vi "01 Maintenance.vi"() -> ()   [LabVIEW 2025]
doc: "This vi provides template for the front panel size fixing for GUI developement."
uses:
  Controls/Maintenance AO Cluster.ctl
  Host Globals/Global 1.vi
  <vilib>/FPGAPlugInAG/Dynamic/niLvFpga_Abort_Dynamic.vi
  <vilib>/FPGAPlugInAG/Dynamic/niLvFpga_Close_Dynamic.vi
  <vilib>/Utility/xml.llb/Read From XML File(string).vi
  <vilib>/rvi/interface/nirviMethod/nirviMethod.xnode
  <vilib>/rvi/interface/nirviCloseFPGA/nirviCloseFPGA.xnode
  <vilib>/rvi/interface/nirviOpenFPGA/nirviOpenFPGA.xnode
  <vilib>/FPGAPlugInAG/Dynamic/niLvFpga_Reset_Dynamic.vi
  <vilib>/FPGAPlugInAG/Dynamic/niLvFpga_Run_Dynamic.vi
  <vilib>/rvi/interface/nirviReadWriteControl/nirviReadWriteControl.xnode
  <vilib>/rvi/interface/Simulation/niFpgaSimulationCallBeginRW.vi
  <vilib>/rvi/errors/niLvFpgaAdjustHostInterfaceError.vi
  FPGA Bitfiles/old.lvbitx
  FPGA Bitfiles/oldMAINFPGANI9148_MKQg3WTXJXE.lvbitx
  NiFpgaLv.dll
panel:
  in  "Misc_P 2":T1={"Gain"=1.0, "offset"=0.0}
  in  "Intercooler_Out_P 2":T1={"Gain"=1.0, "offset"=0.0}
  in  "Intercooler_In_P 2":T1={"Gain"=1.0, "offset"=0.0}
  in  "Oil_P 2":T1={"Gain"=1.0, "offset"=0.0}
  in  "Exhaust_P 2":T1={"Gain"=1.0, "offset"=0.0}
  in  "Coolant_Out_P 2":T1={"Gain"=1.0, "offset"=0.0}
  in  "Coolant_In_P 2":T1={"Gain"=1.0, "offset"=0.0}
  out "Time":string
  out "User":string
  in  "Home Button":bool
  in  "Home":bool caption="Back"
  in  "Tab Control":T2(tab)
  in  "AO Cluster":T3
  in  "4":cluster{"Offset":dbl, "Gain":dbl}
  in  "6":cluster{"Offset":dbl, "Gain":dbl}
  in  "5":cluster{"Offset":dbl, "Gain":dbl}
  in  "2":cluster{"Offset":dbl, "Gain":dbl}
  in  "3":cluster{"Offset":dbl, "Gain":dbl}
  out "ANALOG INPUT":string[][](table)=[["5"], ["1"], ["2.5"], ["5"], ["85"], ["55"], ["7"], ["2"], ["4"], ["2"], ["4"], ["2"], ["5"], ["12.5"], ["22.5"], ["5.02"], ["22.8"], ["7"], ["5"], ["0"], ["0"], ["0.00"], ["0.2"], ["0.1"], ["0.2"]]
  in  "1":cluster{"Offset":dbl, "Gain":dbl}
  in  "DO Cluster":T4
  out "DI Cluster":T5
  # "MAINTENANCE"
  # "Parameters Name"
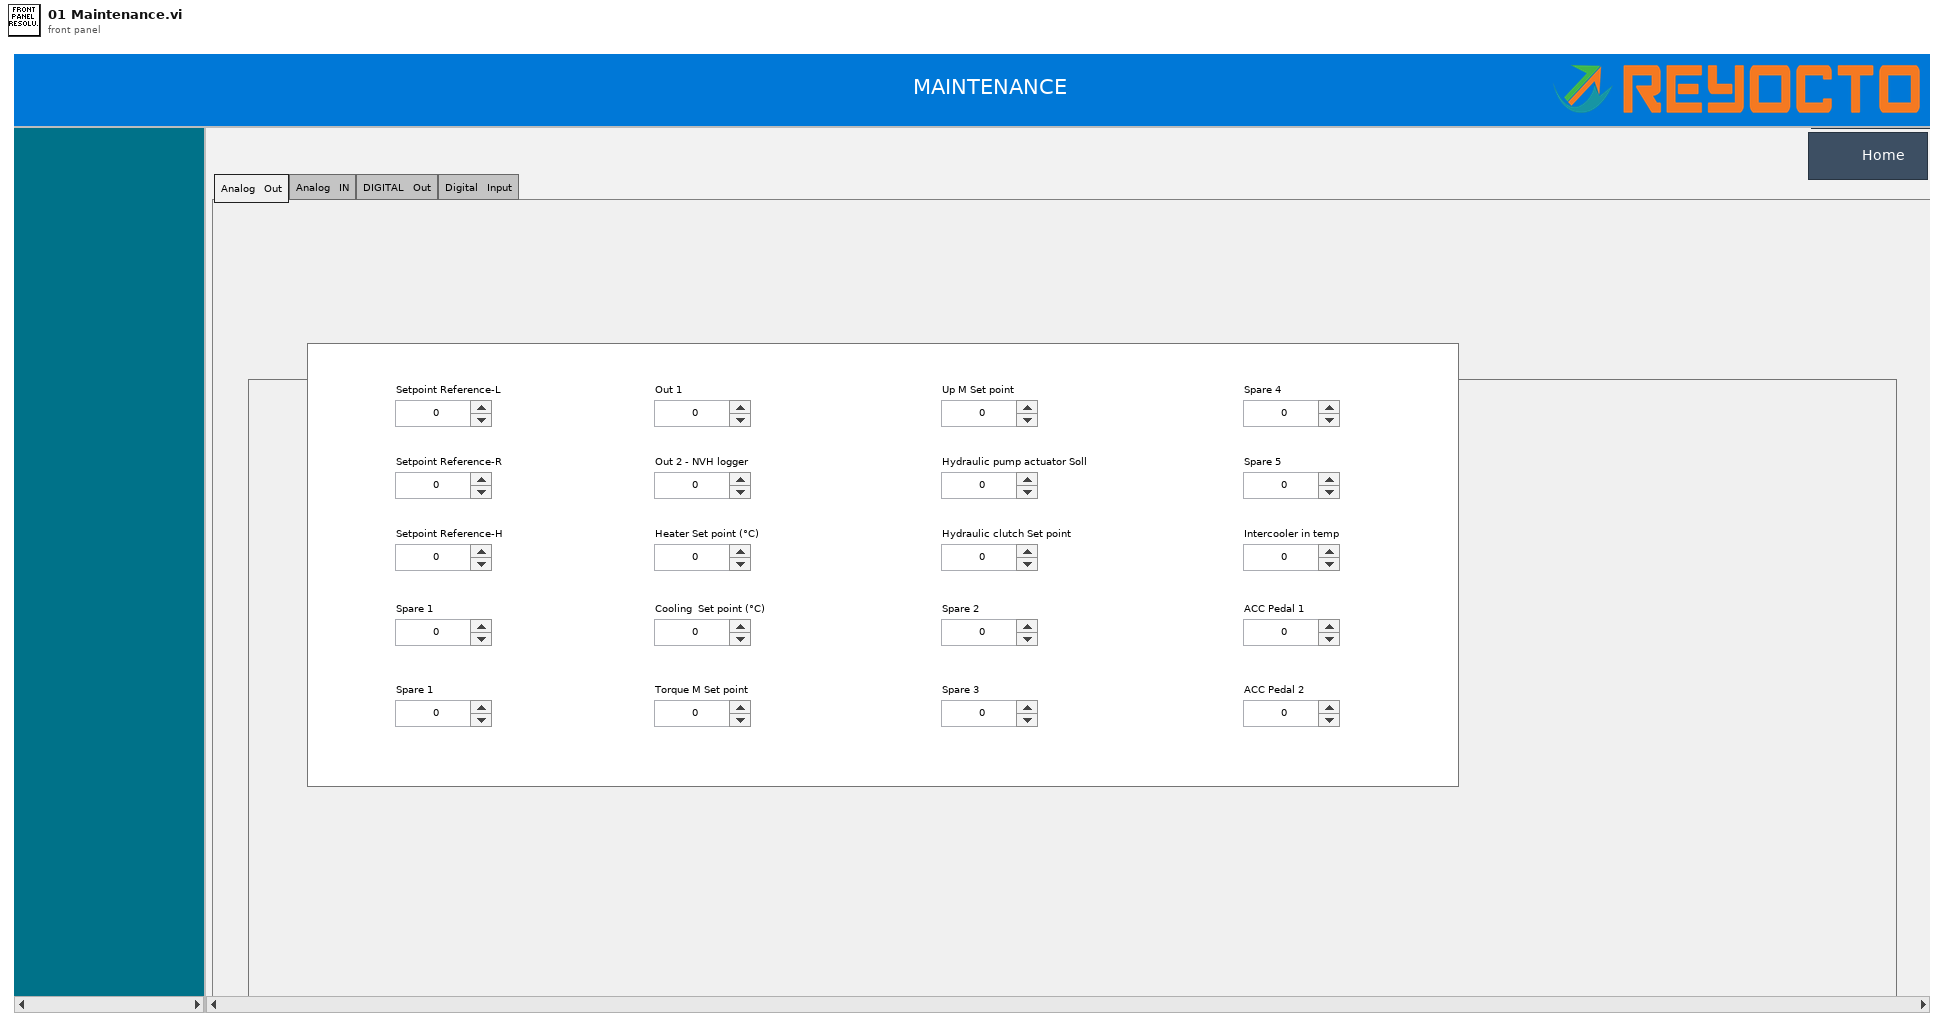
[diagram p1: front panel]
types:
  T1 = cluster{"Gain":fxp<+/-,24,5>, "offset":fxp<+/-,24,5>}
  T2 = enum32{"Analog   Out", "Analog   IN", "DIGITAL   Out", "Digital   Input"}
  T3 = typedef "Maintenance AO Cluster.ctl" = cluster{"AO 1":dbl, "AO 2":dbl, "AO 3":dbl, "AO 4":dbl, "AO 5":dbl, "AO 6":dbl, "AO 7":dbl, "AO 8":dbl, "AO 9":dbl, "AO 10":dbl, "AO 11":dbl, "AO 12":dbl, "AO 13":dbl, "AO 14":dbl, "AO 15":dbl, "AO 16":dbl, "AO 17":dbl, "AO 18":dbl, "AO 19":dbl, "AO 20":dbl}
  T4 = cluster{"0":bool, "1":bool, "2":bool, "3":bool, "4":bool, "5":bool, "6":bool, "7":bool, "8":bool, "9":bool, "10":bool, "11":bool, "12":bool, "13":bool, "14":bool, "15":bool, "16":bool, "17":bool, "18":bool, "19":bool, "20":bool, "21":bool, "22":bool, "23":bool, "24":bool, "25":bool, "26":bool, "27":bool, "28":bool, "29":bool, "30":bool, "31":bool, "32":bool, "33":bool, "34":bool, "35":bool, "36":bool, "37":bool, "38":bool, "39":bool, "40":bool, "41":bool, "42":bool, "43":bool, "44":bool, "45":bool, "46":bool, "47":bool, "48":bool, "49":bool, "50":bool, "51":bool, "52":bool, "53":bool, "54":bool, "55":bool, "56":bool, "57":bool, "58":bool, "59":bool, "60":bool, "61":bool, "62":bool, "63":bool}
  T5 = cluster{"1":bool, "2":bool, "3":bool, "4":bool, "5":bool, "6":bool, "7":bool, "8":bool, "9":bool, "10":bool, "11":bool, "12":bool, "13":bool, "14":bool, "15":bool, "16":bool, "17":bool, "18":bool, "19":bool, "20":bool, "21":bool, "22":bool, "23":bool, "24":bool, "25":bool, "26":bool, "27":bool, "28":bool, "29":bool, "30":bool, "31":bool, "32":bool, "33":bool, "34":bool, "35":bool, "36":bool, "37":bool, "38":bool, "39":bool, "40":bool, "41":bool, "42":bool, "43":bool, "44":bool, "45":bool, "46":bool, "47":bool, "48":bool, "49":bool, "50":bool, "51":bool, "52":bool, "53":bool, "54":bool, "55":bool, "56":bool, "57":bool, "58":bool, "59":bool, "60":bool, "61":bool, "62":bool, "63":bool, "64":bool}
  T6 = enum32{"invalid app kind", "Development System", "Run Time System", "Student Edition", "Embedded LabVIEW", "Evaluation", "Custom"}
  T7 = enum32{"Invalid", "Standard", "Closed", "Hidden", "Minimized", "Maximized"}
  T8 = cluster{"Core":cluster{"Current VI Reference":refnum<vi>, "Close Panel on Exit?":bool}, "AI Config path":path, "AO Config path":path, "DI Config path":path, "DO COnfig path":path, "AO Cluster":refnum<vi>, "DO Cluster":refnum<vi>, "DI Cluster":refnum<vi>, "Data":cluster{"Digital Output":refnum<k21>, "Set 1 DO":u32, "Maintenance":refnum<k21>, "Digital Input":refnum<k21>}, "Analog Data":string[][], "FPGA VI Reference Out":refnum<k20>, "FPGA VI Reference Out":refnum<k20>}
  T9 = cluster{"Digital Output":refnum<k21>, "Set 1 DO":u32, "Maintenance":refnum<k21>, "Digital Input":refnum<k21>}
  T10 = cluster{"Current VI Reference":refnum<vi>, "Close Panel on Exit?":bool}
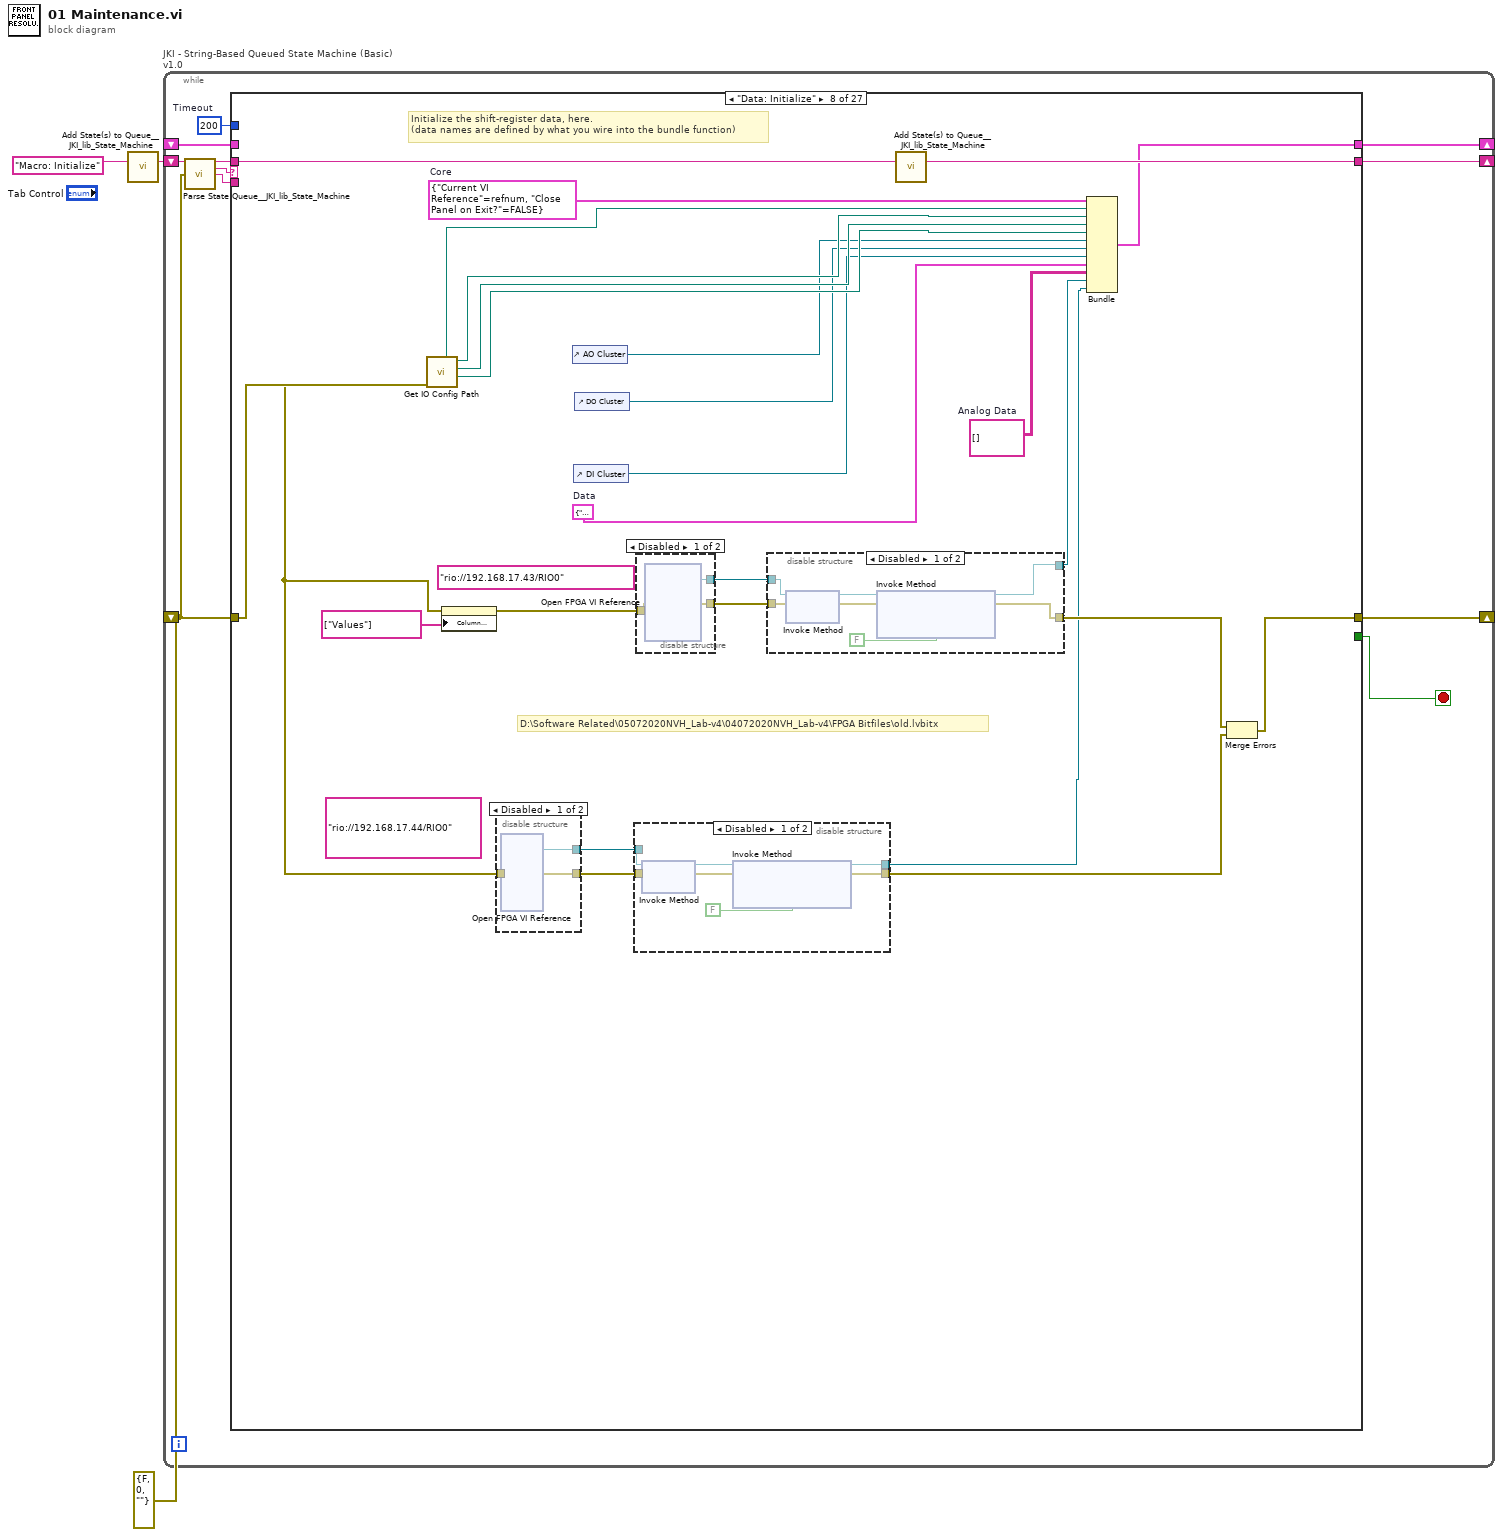
[diagram p0: block diagram]
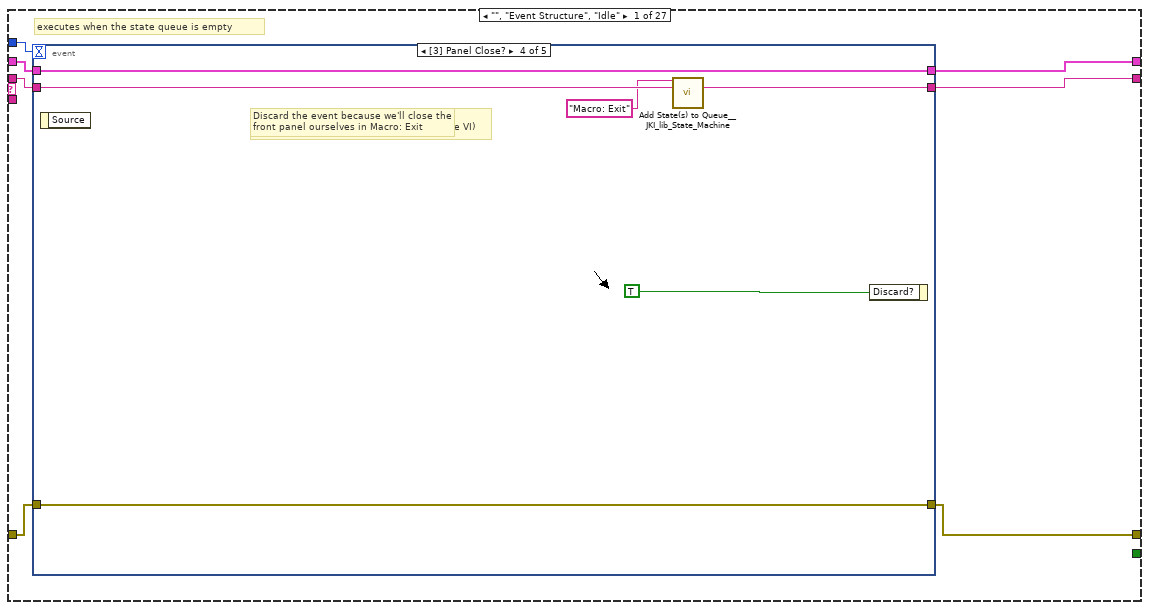
[diagram p2: hidden frame]
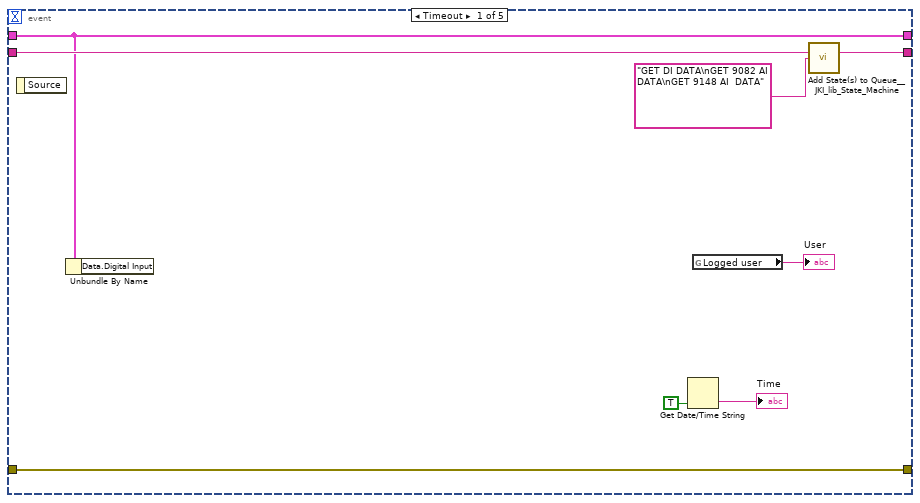
[diagram p3: hidden frame]
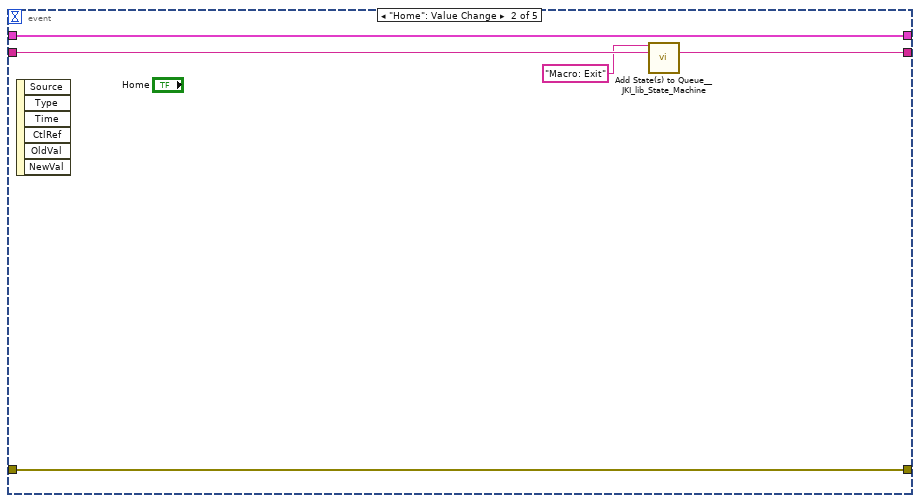
[diagram p4: hidden frame]
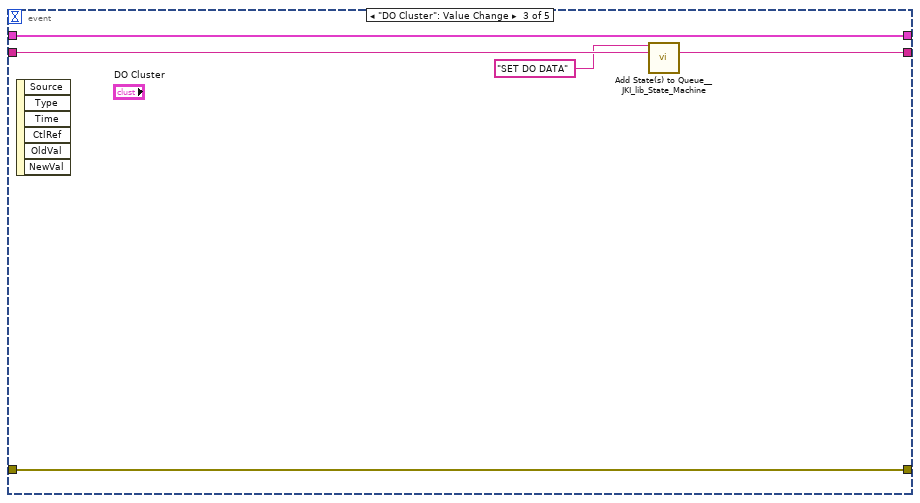
[diagram p5: hidden frame]
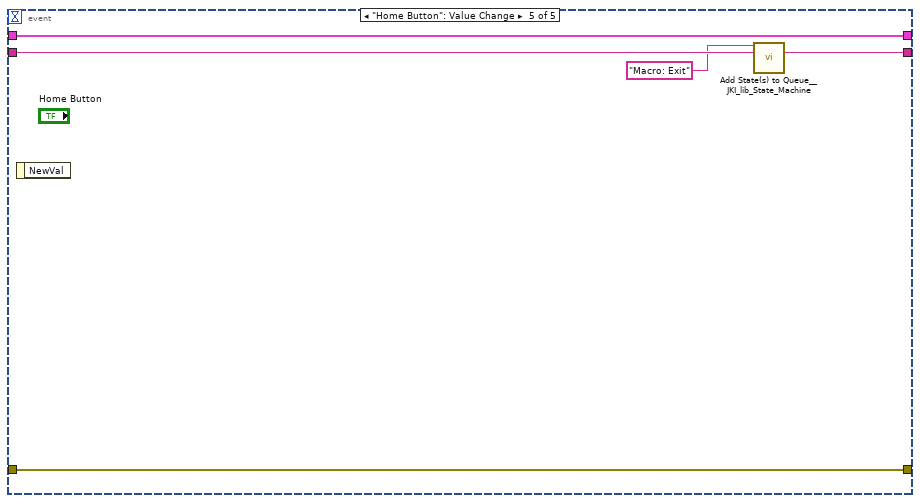
[diagram p6: hidden frame]
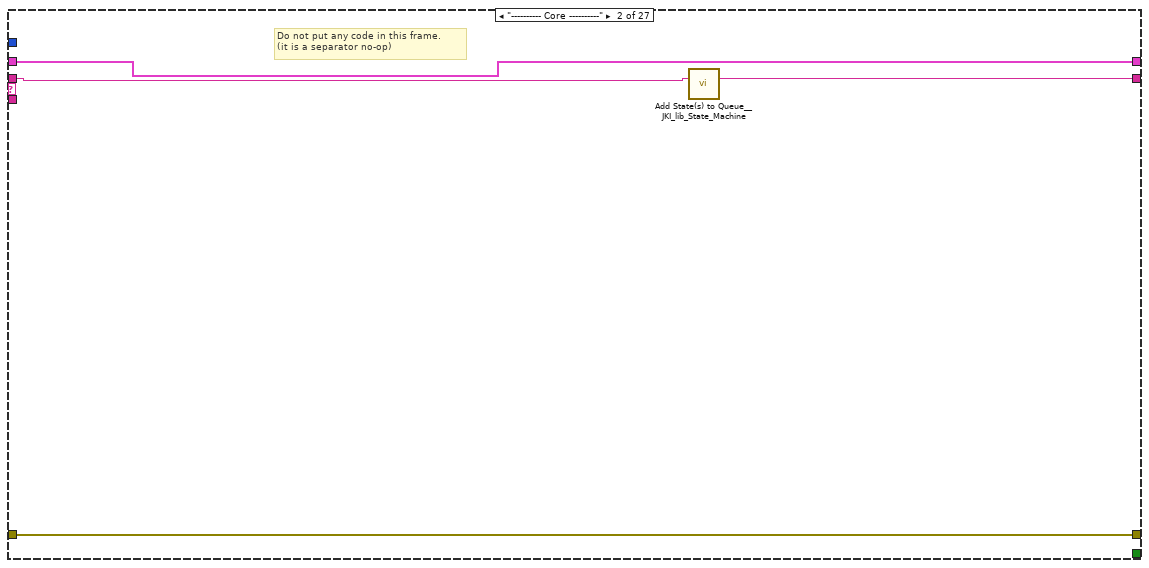
[diagram p7: hidden frame]
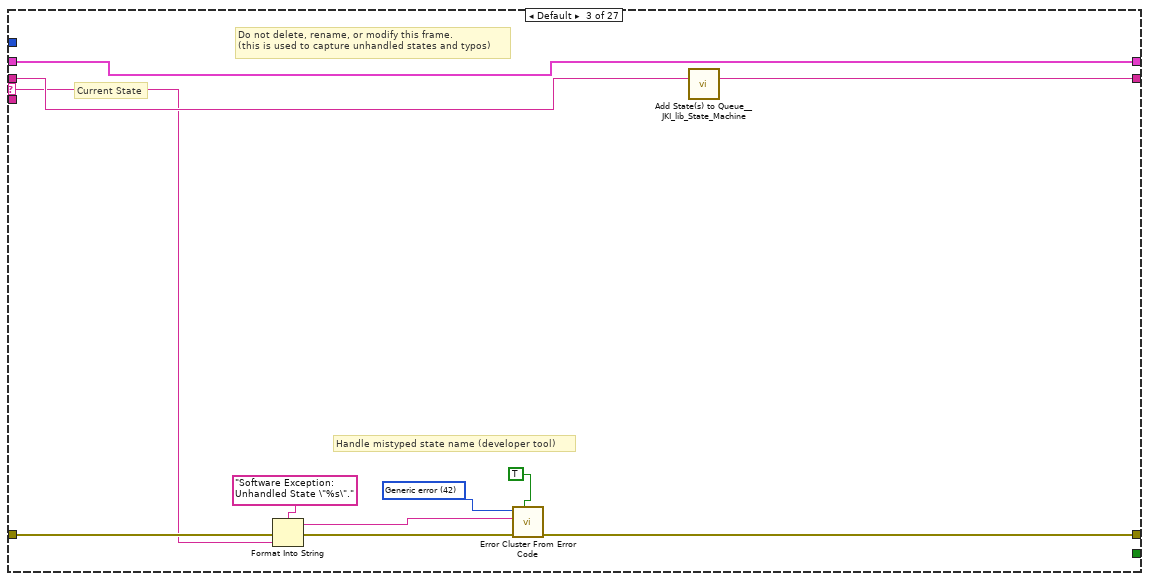
[diagram p8: hidden frame]
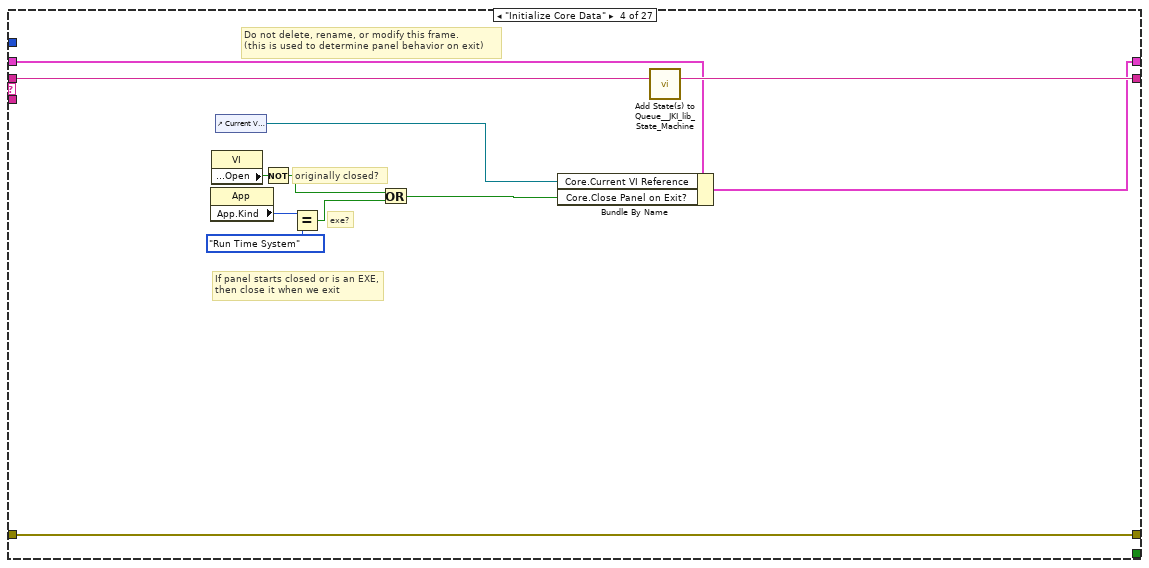
[diagram p9: hidden frame]
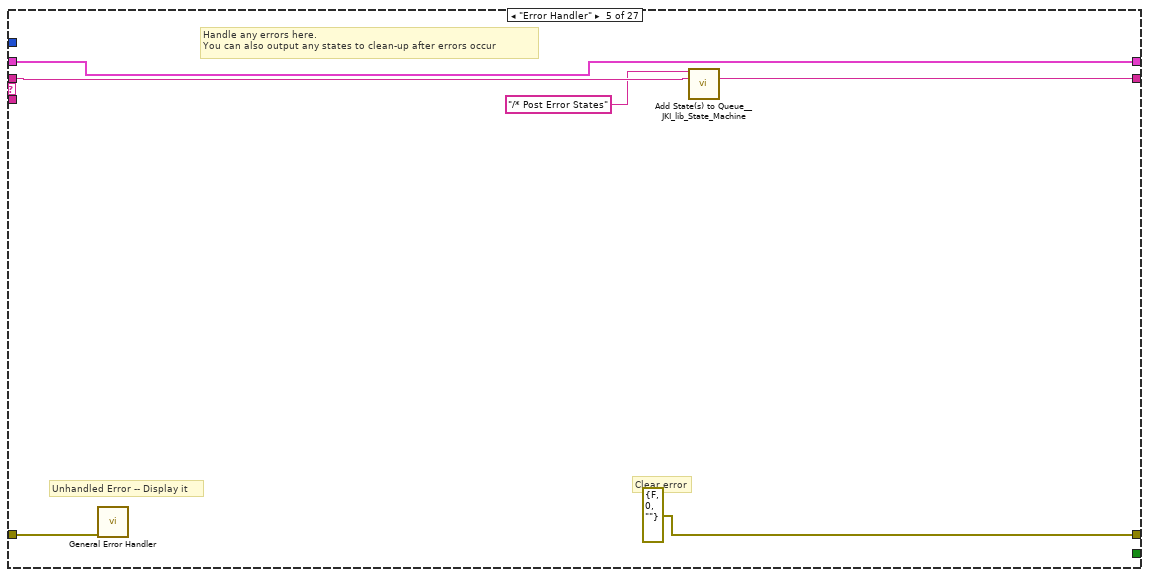
[diagram p10: hidden frame]
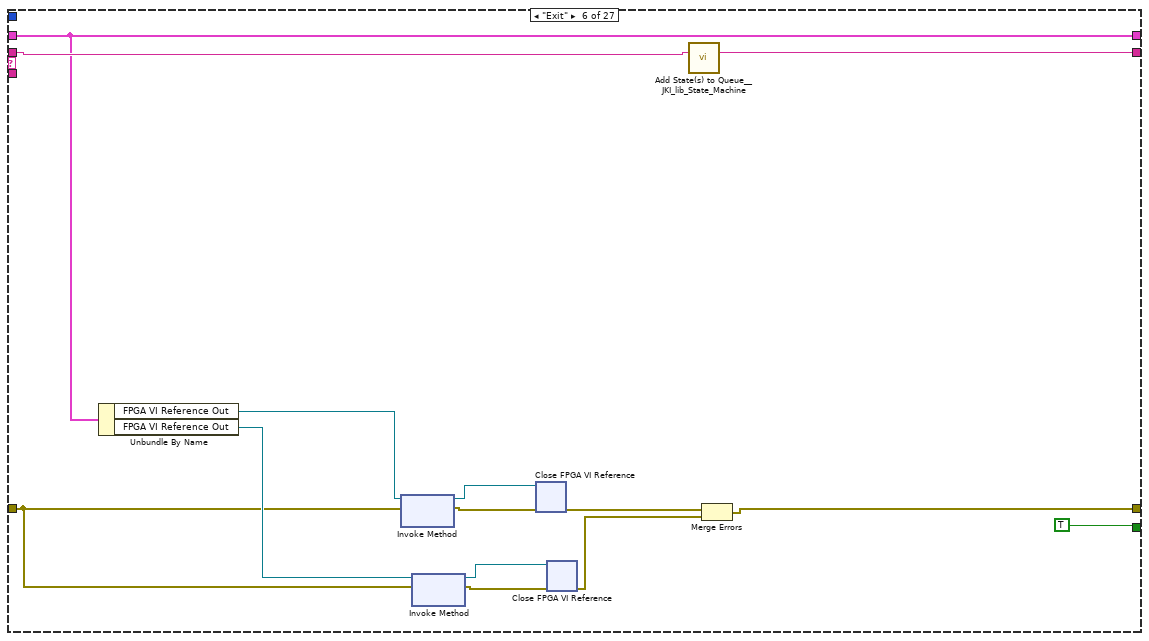
[diagram p11: hidden frame]
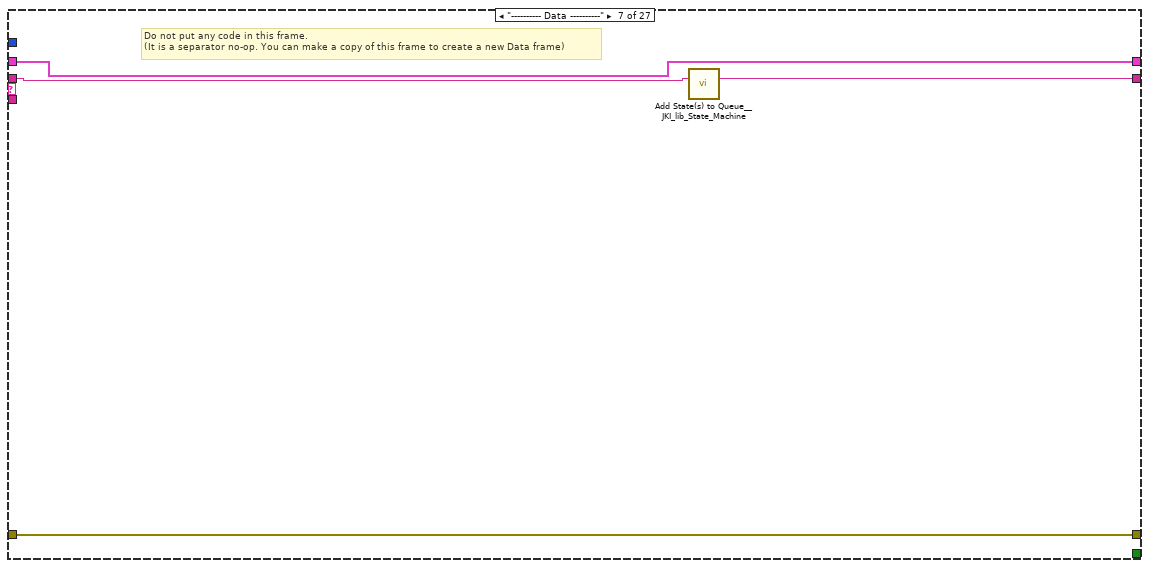
[diagram p12: hidden frame]
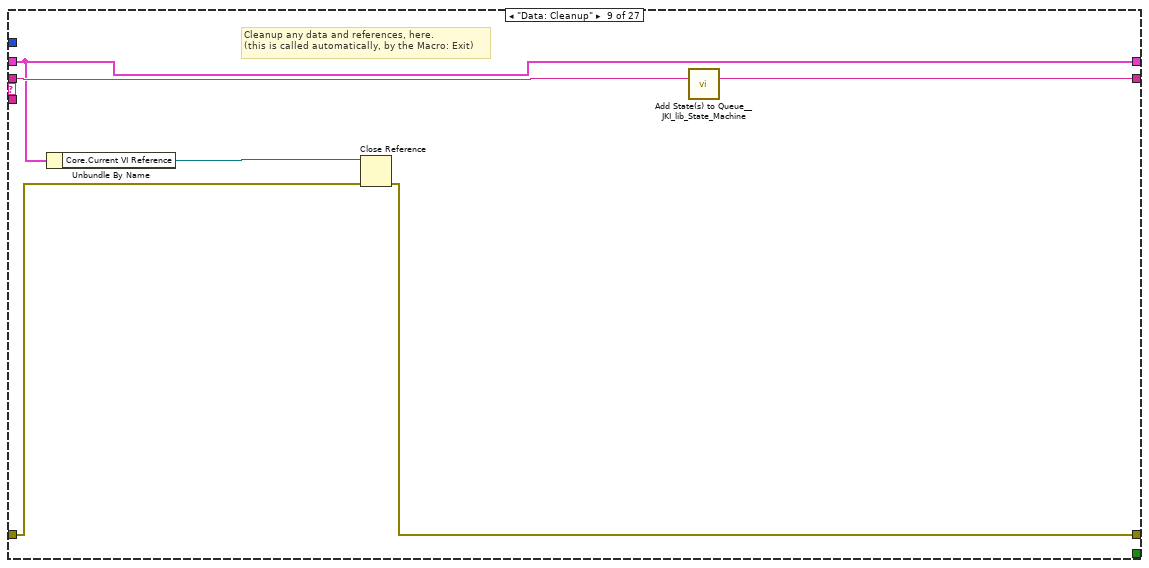
[diagram p17: hidden frame]
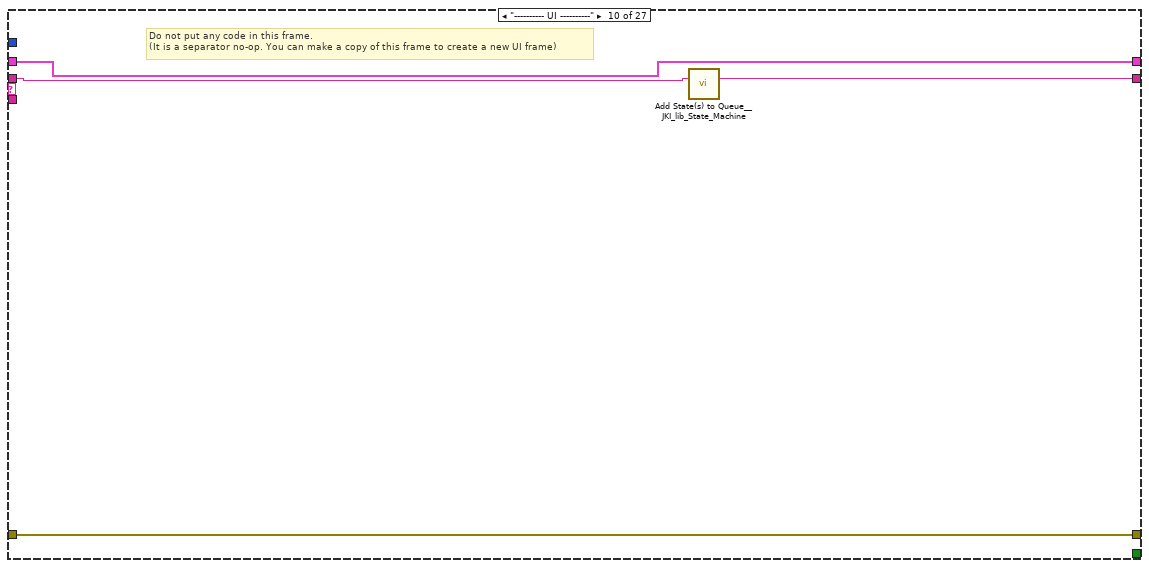
[diagram p18: hidden frame]
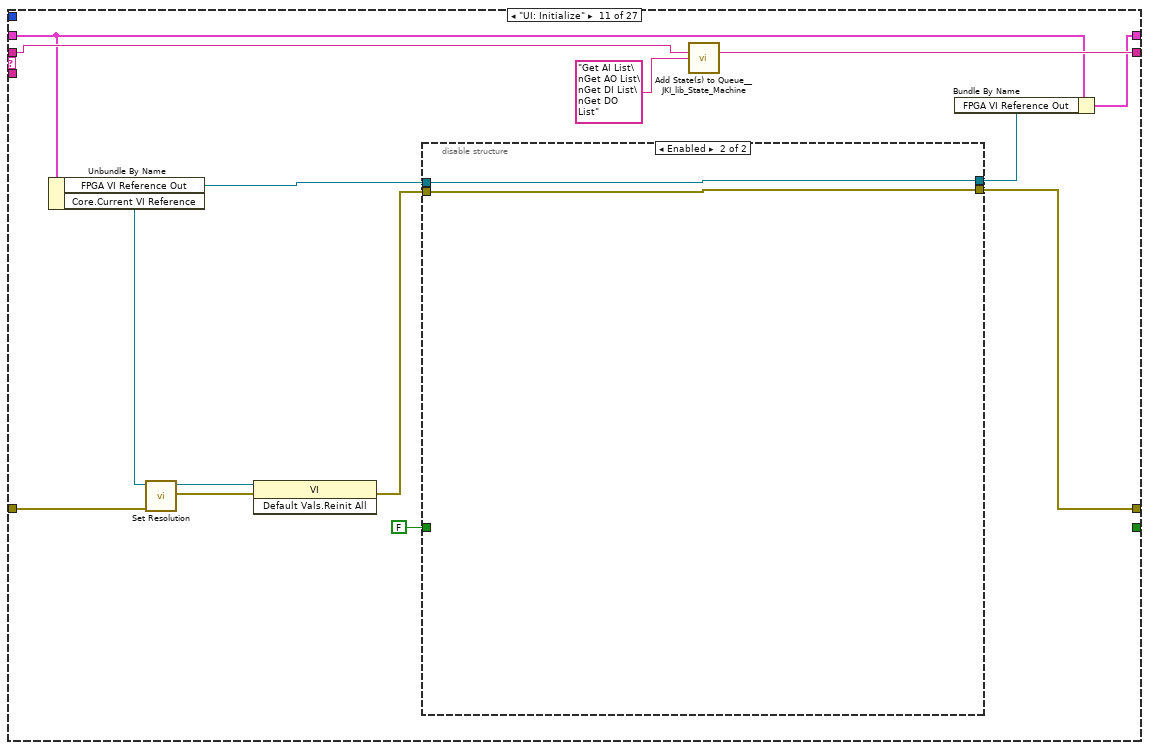
[diagram p19: hidden frame]
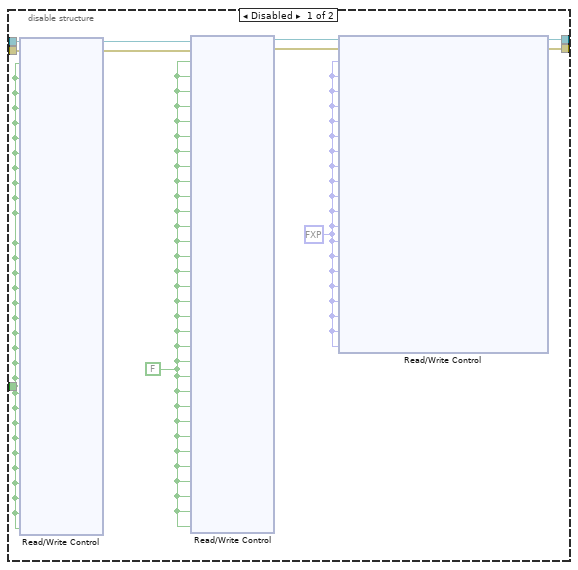
[diagram p20: hidden frame]
diagram:
  n1 = call <vilib>:"Add State(s) to Queue__JKI_lib_State_Machine.vi"("State(s) in (\"\")"="Macro: Initialize") -> ("States Out"=w2:string)  [unwired: 14 in]
  n2 = while "JKI - String-Based Queued State Machine (Basic) v1.0" {
    shift-right: [w7] -> _
    shift-left: _ -> [w6]
    shift-right: [w10] -> _
    shift-left: errorcluster {"status"=FALSE, "code"=0, "source"=""} ("error out") -> [w4]
    shift-right: [w9] -> _
    shift-left: w2 -> [w11]
    stop <- w8 stop-if-true
    w5 = 200  # Timeout
    n3 = call <vilib>:"Parse State Queue__JKI_lib_State_Machine.vi"("State Queue"=w11, "Error In (no error)"=w4) -> ("Remaining States"=w13:string, "Current State"=w14:string, "Arguments"=w12:string)  [unwired: 11 in]
    n4 = case shown="\"Data: Initialize\"" w14 {
      selector: w14 -> [_ _ w55 _ _ _ _ _ _ _ _ _ _ _ _ _ _ _ _ _ _ _ _ _ _ _ _]
      tunnel: w13 -> [w21 w54 w59 w77 w83 w97 w101 w127 w159 w163 w177 w203 w219 w239 w259 w269 w280 w306 w311 w327 w343 w354 w454 w481 w490 w571 w612]
      tunnel: w12 -> [_ _ _ _ _ _ _ _ _ _ _ _ _ _ _ w264 w274 _ _ _ _ _ _ _ _ _ _]
      tunnel: w6 -> [w19 w51 w57 w68 w80 w92 w98 _ w154 w160 w166 w201 w217 w237 w257 w267 w276 w303 w308 w325 w344 w351 w452 w483 w489 w569 w611]
      tunnel: [w18 w52 w61 w74 errorcluster {"status"=FALSE, "code"=0, "source"=""} ("error out") w84 w99 w107 w155 w161 w167 w191 w204 w224 w244 w265 w277 w304 w309 w313 w342 w347 w448 w482 w485 w566 w606] -> w10
      tunnel: w4 -> [w17 w52 w60 w74 w79 w87 w99 w112 w156 w161 w171 w199 w215 w235 w255 w266 w278 w304 w309 w316 w342 w348 w449 w482 w486 w567 w608]
      tunnel: [w20 w53 w58 w76 w82 w96 w100 w126 w158 w162 w176 w202 w218 w238 w258 w268 w279 w305 w310 w326 w343 w353 w454 w481 w490 w571 w612] -> w9
      tunnel: [_ _ _ _ _ TRUE _ _ _ _ _ _ _ _ _ _ _ _ _ _ _ _ _ _ _ _ _] -> w8
      tunnel: [w16 w51 w57 w75 w80 w92 w98 w125 w154 w160 w164 w201 w217 w237 w257 w267 w276 w303 w308 w325 w344 w350 w453 w483 w488 w564 w610] -> w7
      tunnel: w5 -> [w15 _ _ _ _ _ _ _ _ _ _ _ _ _ _ _ _ _ _ _ _ _ _ _ _ _ _]
      frame "", "Event Structure", "Idle" {
        # "executes when the state queue is empty"
        n5 = event shown="[3] Panel Close?" {
          selector: _ -> [_ _ _ _ _]
          dyn-events: _ -> [_ _ _ _ _]
          timeout: w15 -> [_ _ _ _ _]
          tunnel: w21 -> [w29 w34 w39 w45 w47]
          tunnel: [w28 w33 w38 w44 w48] -> w20
          tunnel: w19 -> [w27 w31 w36 w42 w49]
          tunnel: [w23 w32 w37 w43 w50] -> w18
          tunnel: w17 -> [w23 w32 w37 w43 w50]
          tunnel: [w27 w31 w36 w42 w49] -> w16
          event Timeout {
            n6 = event-data() -> ()  [unwired: 1 in, 1 out]
            n7 = Unbundle By Name(w27) -> ()  [unwired: 1 out]
            n8 = Get Date/Time String(want seconds? (F)=TRUE) -> (time string=→"Time":string)  [unwired: 2 in, 1 out]
            n9 = global read "Global 1.vi" "Logged user"() -> (→"User":string)
            n10 = call <vilib>:"Add State(s) to Queue__JKI_lib_State_Machine.vi"("State(s) in (\"\")"=w29, "State(s) at Back (\"\")"="GET DI DATA\nGET 9082 AI  DATA\nGET 9148 AI  DATA" ("State(s) at Back (\"\")")) -> ("States Out"=w28:string)  [unwired: 13 in]
          }
          event "Home": Value Change {
            n11 = event-data() -> ()  [unwired: 1 in, 6 out]
            n12 = call <vilib>:"Add State(s) to Queue__JKI_lib_State_Machine.vi"("State(s) in Front (\"\")"="Macro: Exit", "State(s) in (\"\")"=w34) -> ("States Out"=w33:string)  [unwired: 13 in]
          }
          event "DO Cluster": Value Change {
            n13 = event-data() -> ()  [unwired: 1 in, 6 out]
            n14 = call <vilib>:"Add State(s) to Queue__JKI_lib_State_Machine.vi"("State(s) in Front (\"\")"="SET DO DATA", "State(s) in (\"\")"=w39) -> ("States Out"=w38:string)  [unwired: 13 in]
          }
          event Panel Close? {
            # "Discard the event because we'll close the front panel ourselves in Macro: Exit"
            # "Close Panel button (pressed) Event\n(this executes Macro: Exit to terminate the VI)"
            n15 = event-data() -> ()  [unwired: 1 in, 1 out]
            n16 = call <vilib>:"Add State(s) to Queue__JKI_lib_State_Machine.vi"("State(s) in Front (\"\")"="Macro: Exit", "State(s) in (\"\")"=w45) -> ("States Out"=w44:string)  [unwired: 13 in]
            n17 = event-data("Discard?"=TRUE) -> ()  [unwired: 1 in, 1 out]
          }
          event "Home Button": Value Change {
            n18 = event-data() -> ()  [unwired: 1 in, 1 out]
            n19 = call <vilib>:"Add State(s) to Queue__JKI_lib_State_Machine.vi"("State(s) in Front (\"\")"="Macro: Exit" ("State(s) in Front (\"\")"), "State(s) in (\"\")"=w47) -> ("States Out"=w48:string)  [unwired: 13 in]
          }
        }
      }
      frame "---------- Core ----------" {
        # "Do not put any code in this frame.\n(it is a separator no-op)"
        n20 = call <vilib>:"Add State(s) to Queue__JKI_lib_State_Machine.vi"("State(s) in (\"\")"=w54) -> ("States Out"=w53:string)  [unwired: 14 in]
      }
      frame Default {
        w64 = 42 items=["No error", "Argument error", "Memory is full", "Out of zone", "End of file", "File already open", "Generic file I/O error", "File not found", "File permission error", "Disk is full", "Duplicate path", "Too many files open", "System feature not enabled", "Resource file not found", "Cannot add resource", "Resource not found", "Image not found", "Image memory error", "Pen does not exist", "Config type invalid", "Config token not found", "Config parse error", "Config memory error", "Bad external code format", "Bad external code offset", "External code not present", "Null window", "Destroy window error", "Null menu", "Print aborted", "Bad print record", "Print driver error", "Windows error during printing", "Memory error during printing", "Print dialog error", "Generic print error", "Invalid device refnum", "Device not found", "Device parameter error", "Device unit error", "Cannot open device", "Device call aborted", "Generic error", "Cancelled by user", "Object ID too low", "Object ID too high", "Object not in heap", "Unknown heap", "Unknown object (invalid DefProc)", "Unknown object (DefProc not in table)", "Message out of range", "Invalid (null) method", "Unknown message", "Manager call not supported", "Bad address", "Network operation in progress", "Network operation timed out", "Connection is busy", "Network attribute not supported", "Network error", "Address in use", "System out of memory", "Connection aborted", "Connection refused", "Not connected", "Already connected", "Connection closed", "Initialization error (interapplication manager)", "Bad occurrence", "Wait on unbound occurrence handler", "Occurrence queue overflow", "Datalog type conflict", "Unused", "Unrecognized type (interapplication manager)", "Memory corrupt", "Failed to make temporary DLL", "Old CIN version", "Drag socket not found", "Failed to load drop-object", "Failed to register OLE object", "Failed to release OLE object", "Format specifier type mismatch", "Unknown format specifier", "Too few format specifiers", "Too many format specifiers", "Scan failed", "Newer CIN version", "Error converting to variant", "Runtime menu error", "Password tampered", "Variant attribute not found", "Incompatible variant data type", "Event data is not available", "Event Store is not present", "Occurrence is not found", "Event Queue is not created", "Event info is not available", "Refnum passed is NULL", "Error retrieving Class GUID", "Error retrieving CoClass GUID", "Error retrieving TypeLib GUID.", "Bad built application magic bytes.", "Specific driver is different from the specific driver associated with the Logical Name.", "There is no session opened to the class driver.", "Max Error", "MAX - Error with config objects", "MAX - Error loading configuration", "MAX - Group not supported"]
        # "Current State"
        # "Do not delete, rename, or modify this frame.\n(this is used to capture unhandled states and typos)"
        # "Handle mistyped state name (developer tool)"
        n21 = Format Into String(format string="Software Exception: Unhandled State \"%s\"." ("message"), error in=w60, w55) -> (resulting string=w63:string, error out=w62:errorcluster)  [unwired: 1 in]
        n22 = call <vilib>:"Error Cluster From Error Code.vi"("show call chain? (False)"=TRUE, "error in (no error)"=w62, "error message (\"\")"=w63, "error code (0)"=w64) -> ("error out"=w61:errorcluster)  [unwired: 5 in]
        n23 = call <vilib>:"Add State(s) to Queue__JKI_lib_State_Machine.vi"("State(s) in (\"\")"=w59) -> ("States Out"=w58:string)  [unwired: 14 in]
      }
      frame "Initialize Core Data" {
        # "Do not delete, rename, or modify this frame.\n(this is used to determine panel behavior on exit)"
        # "originally closed?"
        # "exe?"
        # "If panel starts closed or is an EXE, then close it when we exit"
        n24 = property class="App"() -> ("App.Kind"=w72:T6)  [unwired: 2 in, 2 out]
        n25 = property class="VI"() -> ("Front Panel.Open"=w73:bool)  [unwired: 2 in, 2 out]
        n26 = control-ref of="Current VI Reference"() -> (w66:refnum<vi>)
        n27 = Not(x=w73) -> (.not. x?=w70:bool)
        n28 = Equal?(x=w72, y=T6."Run Time System" ("Application:Kind")) -> (x = y?=w69:bool)
        n29 = Or(x=w70, y=w69) -> (x .or. y?=w67:bool)
        n30 = Bundle By Name(cluster=w68, "Core.Current VI Reference"=w66, "Core.Close Panel on Exit?"=w67) -> (w75:T8)
        n31 = call <vilib>:"Add State(s) to Queue__JKI_lib_State_Machine.vi"("State(s) in (\"\")"=w77) -> ("States Out"=w76:string)  [unwired: 14 in]
      }
      frame "Error Handler" {
        # "Unhandled Error -- Display it"
        # "Handle any errors here.\nYou can also output any states to clean-up after errors occur"
        # "Clear error"
        n32 = call <vilib>:"General Error Handler.vi"("error in (no error)"=w79) -> ()  [unwired: 10 in, 5 out]
        n33 = call <vilib>:"Add State(s) to Queue__JKI_lib_State_Machine.vi"("State(s) in Front (\"\")"="/* Post Error States", "State(s) in (\"\")"=w83) -> ("States Out"=w82:string)  [unwired: 13 in]
      }
      frame "Exit" {
        n34 = Unbundle By Name(w92) -> ("FPGA VI Reference Out"=w91:refnum<k20>, "FPGA VI Reference Out"=w88:refnum<k20>)
        n35 = xnode "Invoke Method"("FPGA VI Reference In"=w91, "error in"=w87) -> ("FPGA VI Reference Out"=w93:refnum<k20>, "error out"=w94:errorcluster)
        n36 = xnode "Invoke Method"("FPGA VI Reference In"=w88, "error in"=w87) -> ("FPGA VI Reference Out"=w90:refnum<k20>, "error out"=w89:errorcluster)
        n37 = xnode "Close FPGA VI Reference"("FPGA VI Reference In"=w93, "error in"=w94) -> ("error out"=w85:errorcluster)
        n38 = xnode "Close FPGA VI Reference"("FPGA VI Reference In"=w90, "error in"=w89) -> ("error out"=w86:errorcluster)
        n39 = call <vilib>:"Add State(s) to Queue__JKI_lib_State_Machine.vi"("State(s) in (\"\")"=w97) -> ("States Out"=w96:string)  [unwired: 14 in]
        n40 = Merge Errors(w85, w86) -> (w84:errorcluster)
      }
      frame "---------- Data ----------" {
        # "Do not put any code in this frame.\n(It is a separator no-op. You can make a copy of this frame to create a new Data frame)"
        n41 = call <vilib>:"Add State(s) to Queue__JKI_lib_State_Machine.vi"("State(s) in (\"\")"=w101) -> ("States Out"=w100:string)  [unwired: 14 in]
      }
      frame "Data: Initialize" {
        w103 = string[][] []  # Analog Data
        (unwired) tag "rio://192.168.17.44/RIO0" ("resource name")
        (unwired) tag "rio://192.168.17.43/RIO0" ("resource name")
        w123 = T9 {"Digital Output"="", "Set 1 DO"=0, "Maintenance"="", "Digital Input"=""}  # Data
        w124 = T10 {"Current VI Reference"=refnum, "Close Panel on Exit?"=FALSE}  # Core
        # "D:\\Software Related\\05072020NVH_Lab-v4\\04072020NVH_Lab-v4\\FPGA Bitfiles\\old.lvbitx"
        # "Initialize the shift-register data, here.\n(data names are defined by what you wire into the bundle function)"
        n42 = call "Get IO Config Path.vi"("error in (no error)"=w112) -> ("error out"=w105:errorcluster, "DO COnfig path"=w119:path, "DI Config path"=w120:path, "AO Config path"=w121:path, "AI Config path"=w122:path)  [unwired: 5 in, 1 out]
        n43 = property on="ANALOG INPUT" class="Tbl (strict)"(error in=w105, "Column Headers[]"=string[] ["Values"] ("Row Header Strings[]")) -> (error out=w104:errorcluster)  [unwired: 1 in, 1 out]
        n44 = disable-structure shown="Disabled" {
          disable-tunnel: [w148 _] -> w111
          disable-tunnel: [w147 w149] -> w110
          disable-tunnel: w105 -> [w146 w149]
          frame Disabled {
            n45 = xnode "Open FPGA VI Reference"("error in"=w146) -> ("FPGA VI Reference Out"=w148:refnum<k20>, "error out"=w147:errorcluster)  [unwired: 1 in]
          }
          frame Enabled {
          }
        }
        n46 = control-ref of="AO Cluster"() -> (w118:refnum<vi>)
        n47 = control-ref of="DI Cluster"() -> (w116:refnum<vi>)
        n48 = control-ref of="DO Cluster"() -> (w117:refnum<vi>)
        n49 = disable-structure shown="Disabled" {
          disable-tunnel: w111 -> [w133 w135]
          disable-tunnel: w110 -> [w132 w136]
          disable-tunnel: [w129 w136] -> w109
          disable-tunnel: [w128 w135] -> w102
          frame Disabled {
            n50 = xnode "Invoke Method"("FPGA VI Reference In"=w133, "error in"=w132) -> ("FPGA VI Reference Out"=w131:refnum<k20>, "error out"=w130:errorcluster)
            n51 = xnode "Invoke Method"("FPGA VI Reference In"=w131, "error in"=w130, "Wait Until Done (F)"=FALSE) -> ("FPGA VI Reference Out"=w128:refnum<k20>, "error out"=w129:errorcluster)
          }
          frame Enabled {
          }
        }
        n52 = disable-structure shown="Disabled" {
          disable-tunnel: [w152 w153] -> w115
          disable-tunnel: [w151 _] -> w114
          disable-tunnel: w104 -> [w150 w153]
          frame Disabled {
            n53 = xnode "Open FPGA VI Reference"("error in"=w150) -> ("FPGA VI Reference Out"=w151:refnum<k20>, "error out"=w152:errorcluster)  [unwired: 1 in]
          }
          frame Enabled {
          }
        }
        n54 = disable-structure shown="Disabled" {
          disable-tunnel: w115 -> [w141 w144]
          disable-tunnel: w114 -> [w140 w145]
          disable-tunnel: [w138 w145] -> w113
          disable-tunnel: [w137 w144] -> w108
          frame Disabled {
            n55 = xnode "Invoke Method"("FPGA VI Reference In"=w140, "error in"=w141) -> ("FPGA VI Reference Out"=w142:refnum<k20>, "error out"=w143:errorcluster)
            n56 = xnode "Invoke Method"("FPGA VI Reference In"=w142, "error in"=w143, "Wait Until Done (F)"=FALSE) -> ("FPGA VI Reference Out"=w138:refnum<k20>, "error out"=w137:errorcluster)
          }
          frame Enabled {
          }
        }
        n57 = call <vilib>:"Add State(s) to Queue__JKI_lib_State_Machine.vi"("State(s) in (\"\")"=w127) -> ("States Out"=w126:string)  [unwired: 14 in]
        n58 = Bundle("Core"=w124, "AI Config path"=w122, "AO Config path"=w121, "DI Config path"=w120, "DO COnfig path"=w119, "AO Cluster"=w118, "DO Cluster"=w117, "DI Cluster"=w116, "Data"=w123, "Analog Data"=w103, "FPGA VI Reference Out"=w113, "FPGA VI Reference Out"=w102) -> (w125:T8)  [unwired: 1 in]
        n59 = Merge Errors(w108, w109) -> (w107:errorcluster)
      }
      frame "Data: Cleanup" {
        # "Cleanup any data and references, here.\n(this is called automatically, by the Macro: Exit)"
        n60 = Unbundle By Name(w154) -> ("Core.Current VI Reference"=w157:refnum<vi>)
        n61 = Close Reference(reference=w157, error in (no error)=w156) -> (error out=w155:errorcluster)
        n62 = call <vilib>:"Add State(s) to Queue__JKI_lib_State_Machine.vi"("State(s) in (\"\")"=w159) -> ("States Out"=w158:string)  [unwired: 14 in]
      }
      frame "---------- UI ----------" {
        # "Do not put any code in this frame.\n(It is a separator no-op. You can make a copy of this frame to create a new UI frame)"
        n63 = call <vilib>:"Add State(s) to Queue__JKI_lib_State_Machine.vi"("State(s) in (\"\")"=w163) -> ("States Out"=w162:string)  [unwired: 14 in]
      }
      frame "UI: Initialize" {
        n64 = Unbundle By Name(w166) -> ("FPGA VI Reference Out"=w169:refnum<k20>, "Core.Current VI Reference"=w175:refnum<vi>)
        n65 = call "Set Resolution.vi"("error in (no error)"=w171, "VI in"=w175) -> ("error out"=w172:errorcluster, "VI out"=w173:refnum<vi>)  [unwired: 8 in]
        n66 = invoke class="VI" method="Default Vals.Reinit All"(reference=w173, error in=w172) -> (error out=w168:errorcluster)  [unwired: 1 in, 2 out]
        n67 = disable-structure shown="Enabled" {
          disable-tunnel: FALSE -> [w187 _]
          disable-tunnel: w169 -> [w186 w189]
          disable-tunnel: w168 -> [w182 w190]
          disable-tunnel: [w179 w190] -> w167
          disable-tunnel: [w178 w189] -> w165
          frame Disabled {
            w183 = FALSE
            w188 = fxp<+/-,20,5> 0.0 ("Mod1/AO0..L")
            n68 = xnode "Read/Write Control"("FPGA VI Reference In"=w186, "error in"=w182, "Mod3/DO0"=w187, "Mod3/DO1"=w187, "Mod3/DO2"=w187, "Mod3/DO3"=w187, "Mod3/DO4"=w187, "Mod3/DO5"=w187, "Mod3/DO6"=w187, "Mod3/DO7"=w187, "Mod3/DO8"=w187, "Mod3/DO9"=w187, "Mod3/DO10"=w187, "Mod3/DO12"=w187, "Mod3/DO13"=w187, "Mod3/DO14"=w187, "Mod3/DO15"=w187, "Mod3/DO16"=w187, "Mod3/DO17"=w187, "Mod3/DO18"=w187, "Mod3/DO19"=w187, "Mod3/DO20"=w187, "Mod3/DO21"=w187, "Mod3/DO22"=w187, "Mod3/DO23"=w187, "Mod3/DO24"=w187, "Mod3/DO25"=w187, "Mod3/DO26"=w187, "Mod3/DO27"=w187, "Mod3/DO28"=w187, "Mod3/DO29"=w187, "Mod3/DO30"=w187, "Mod3/DO31"=w187) -> ("FPGA VI Reference Out"=w185:refnum<k20>, "error out"=w181:errorcluster)  [unwired: 1 in]
            n69 = xnode "Read/Write Control"("FPGA VI Reference In"=w185, "error in"=w181, "Mod3/DO0"=w183, "Mod3/DO1"=w183, "Mod3/DO2"=w183, "Mod3/DO3"=w183, "Mod3/DO4"=w183, "Mod3/DO5"=w183, "Mod3/DO6"=w183, "Mod3/DO7"=w183, "Mod3/DO8"=w183, "Mod3/DO9"=w183, "Mod3/DO10"=w183, "Mod3/DO11"=w183, "Mod3/DO12"=w183, "Mod3/DO13"=w183, "Mod3/DO14"=w183, "Mod3/DO15"=w183, "Mod3/DO16"=w183, "Mod3/DO17"=w183, "Mod3/DO18"=w183, "Mod3/DO19"=w183, "Mod3/DO20"=w183, "Mod3/DO21"=w183, "Mod3/DO22"=w183, "Mod3/DO23"=w183, "Mod3/DO24"=w183, "Mod3/DO25"=w183, "Mod3/DO26"=w183, "Mod3/DO27"=w183, "Mod3/DO28"=w183, "Mod3/DO29"=w183, "Mod3/DO30"=w183, "Mod3/DO31"=w183) -> ("FPGA VI Reference Out"=w184:refnum<k20>, "error out"=w180:errorcluster)
            n70 = xnode "Read/Write Control"("FPGA VI Reference In"=w184, "error in"=w180, "Mod1/AO0..L"=w188, "Mod1/AO0..R"=w188, "Mod1/AO0..H"=w188, "Mod1/AO0..spare"=w188, "Mod7/Spare1"=w188, "Mod7/Out 1"=w188, "Mod7/Out 2"=w188, "Heater Set point (°C)"=w188, "Cooling  Set point (°C)"=w188, "Mod7/Torque M Set point"=w188, "Mod7/Up M Set point"=w188, "Mod7/Hydraulic pump actuator Soll"=w188, "Mod7/Hydraulic clutch Set point"=w188, "Mod7/Spare2"=w188, "Mod7/Spare 3"=w188, "Mod7/Spare 4"=w188, "Mod7/Spare 5"=w188, "Mod7/Spare 6"=w188, "Mod7/Spare 7"=w188, "Mod7/Spare 8"=w188) -> ("FPGA VI Reference Out"=w178:refnum<k20>, "error out"=w179:errorcluster)
          }
          frame Enabled {
          }
        }
        n71 = call <vilib>:"Add State(s) to Queue__JKI_lib_State_Machine.vi"("State(s) in (\"\")"=w177, "State(s) at Back (\"\")"="Get AI List\nGet AO List\nGet DI List\nGet DO List" ("State(s) at Back (\"\")")) -> ("States Out"=w176:string)  [unwired: 13 in]
        n72 = Bundle By Name(cluster=w166, "FPGA VI Reference Out"=w165) -> (w164:T8)
      }
      frame "Get AI List" {
        n73 = Unbundle By Name(w201) -> ("AI Config path"=w200:path)
        n74 = call-poly <vilib>:"Read From XML File.vi"("error in (no error)"=w199, "XML File Path"=w200) -> ("error out"=w196:errorcluster, "XML Elements"=w198:string)  [unwired: 7 in, 1 out]
        n75 = Unflatten From XML(xml string=w198, type=string[][] [], error in (no error)=w196) -> (value=w195:string[][], error out=w192:errorcluster)
        n76 = Index Array(array=w195, index (col)=2 ("disabled index (col)")) -> (element=w193:string[])  [unwired: 1 in]
        n77 = property on="ANALOG INPUT" class="Tbl (strict)"(error in=w192, "Row Headers[]"=w193) -> (error out=w191:errorcluster)  [unwired: 1 in, 1 out]
        n78 = call <vilib>:"Add State(s) to Queue__JKI_lib_State_Machine.vi"("State(s) in (\"\")"=w203) -> ("States Out"=w202:string)  [unwired: 14 in]
      }
      frame "Get AO List" {
        n79 = Unbundle By Name(w217) -> ("AO Cluster"=w209:refnum<vi>, "AO Config path"=w216:path)
        n80 = call-poly <vilib>:"Read From XML File.vi"("error in (no error)"=w215, "XML File Path"=w216) -> ("error out"=w212:errorcluster, "XML Elements"=w214:string)  [unwired: 7 in, 1 out]
        n81 = Unflatten From XML(xml string=w214, type=string[][] [], error in (no error)=w212) -> (value=w211:string[][], error out=w208:errorcluster)
        n82 = Index Array(array=w211, index (col)=2 ("disabled index (col)")) -> (element=w205:string[])  [unwired: 1 in]
        n83 = property class="Clust (strict)"(reference=w209, error in=w208) -> (error out=w206:errorcluster, "Controls[]"=w207:refnum<vi>[])  [unwired: 1 out]
        n84 = for {
          tunnel: w207 -> [w222] mode=indexing
          shift-right: [w221] -> w204
          shift-left: w206 -> [w223]
          tunnel: w205 -> [w220] mode=indexing
          n85 = property class="Ctl"(reference=w222, error in=w223, "Caption.Text"=w220) -> (error out=w221:errorcluster)  [unwired: 1 out]
        }
        n86 = call <vilib>:"Add State(s) to Queue__JKI_lib_State_Machine.vi"("State(s) in (\"\")"=w219) -> ("States Out"=w218:string)  [unwired: 14 in]
      }
      frame "Get DI List" {
        n87 = Unbundle By Name(w237) -> ("DI Cluster"=w229:refnum<vi>, "DI Config path"=w236:path)
        n88 = call-poly <vilib>:"Read From XML File.vi"("error in (no error)"=w235, "XML File Path"=w236) -> ("error out"=w232:errorcluster, "XML Elements"=w234:string)  [unwired: 7 in, 1 out]
        n89 = Unflatten From XML(xml string=w234, type=string[][] [], error in (no error)=w232) -> (value=w231:string[][], error out=w228:errorcluster)
        n90 = Index Array(array=w231, index (col)=2 ("disabled index (col)")) -> (element=w225:string[])  [unwired: 1 in]
        n91 = property class="Clust (strict)"(reference=w229, error in=w228) -> (error out=w226:errorcluster, "Controls[]"=w227:refnum<vi>[])  [unwired: 1 out]
        n92 = for {
          tunnel: w227 -> [w242] mode=indexing
          shift-right: [w241] -> w224
          shift-left: w226 -> [w243]
          tunnel: w225 -> [w240] mode=indexing
          n93 = property class="Ctl"(reference=w242, error in=w243, "Caption.Text"=w240) -> (error out=w241:errorcluster)  [unwired: 1 out]
        }
        n94 = call <vilib>:"Add State(s) to Queue__JKI_lib_State_Machine.vi"("State(s) in (\"\")"=w239) -> ("States Out"=w238:string)  [unwired: 14 in]
      }
      frame "Get DO List" {
        n95 = Unbundle By Name(w257) -> ("DO Cluster"=w249:refnum<vi>, "DO COnfig path"=w256:path)
        n96 = call-poly <vilib>:"Read From XML File.vi"("error in (no error)"=w255, "XML File Path"=w256) -> ("error out"=w252:errorcluster, "XML Elements"=w254:string)  [unwired: 7 in, 1 out]
        n97 = Unflatten From XML(xml string=w254, type=string[][] [], error in (no error)=w252) -> (value=w251:string[][], error out=w248:errorcluster)
        n98 = Index Array(array=w251, index (col)=2 ("disabled index (col)")) -> (element=w245:string[])  [unwired: 1 in]
        n99 = property class="Clust (strict)"(reference=w249, error in=w248) -> (error out=w246:errorcluster, "Controls[]"=w247:refnum<vi>[])  [unwired: 1 out]
        n100 = for {
          tunnel: w247 -> [w262] mode=indexing
          shift-right: [w261] -> w244
          shift-left: w246 -> [w263]
          tunnel: w245 -> [w260] mode=indexing
          n101 = property class="Ctl"(reference=w262, error in=w263, "Caption.Text"=w260) -> (error out=w261:errorcluster)  [unwired: 1 out]
        }
        n102 = call <vilib>:"Add State(s) to Queue__JKI_lib_State_Machine.vi"("State(s) in (\"\")"=w259) -> ("States Out"=w258:string)  [unwired: 14 in]
      }
      frame "UI: Cursor Set" {
        # "Argument"
        # "Set and Unset Cursor Busy.\n(Usage: \"UI: Cursor Set >> Busy|Idle\")"
        n103 = case shown="\"Idle\", Default" w264 {
          tunnel: w266 -> [w271 w273]
          tunnel: [w270 w272] -> w265
          frame "Idle", Default {
            n104 = call <vilib>:"Unset Busy.vi"("error in (no error)"=w271) -> ("error out"=w270:errorcluster)  [unwired: 10 in]
          }
          frame "Busy" {
            n105 = call <vilib>:"Set Busy.vi"("error in (no error)"=w273) -> ("error out"=w272:errorcluster)  [unwired: 9 in, 1 out]
          }
        }
        n106 = call <vilib>:"Add State(s) to Queue__JKI_lib_State_Machine.vi"("State(s) in (\"\")"=w269) -> ("States Out"=w268:string)  [unwired: 14 in]
      }
      frame "UI: Front Panel State" {
        # "Argument"
        # "Set Front Panel Open or Closed\n(Usage: \"UI: Front Panel State >> Open|Close\")"
        n107 = Unbundle By Name(w276) -> ("Core.Current VI Reference"=w275:refnum<vi>)
        n108 = case shown="\"Open\", Default" w274 {
          tunnel: w278 -> [w284 w297]
          tunnel: [w286 w298] -> w277
          tunnel: w275 -> [w285 w295]
          frame "Open", Default {
            n109 = property class="VI"(reference=w285, error in=w284) -> (reference out=w282:refnum<vi>, error out=w283:errorcluster, "Front Panel.Open"=w281:bool)
            n110 = case shown="True" w281 {
              tunnel: [w289 w292] -> w286
              tunnel: w283 -> [w288 w292]
              tunnel: w282 -> [w287 _]
              frame False {
                n111 = invoke class="VI" method="FP.Open"(reference=w287, error in=w288, "Activate"=TRUE, "State"=T7."Standard") -> (error out=w289:errorcluster)  [unwired: 1 in, 4 out]
              }
              frame True {
              }
            }
          }
          frame "Close" {
            n112 = property class="VI"(reference=w295, error in=w297) -> (reference out=w294:refnum<vi>, error out=w296:errorcluster, "Front Panel.Open"=w293:bool)
            n113 = case shown="True" w293 {
              tunnel: [w299 w302] -> w298
              tunnel: w296 -> [w299 w301]
              tunnel: w294 -> [_ w300]
              frame False {
              }
              frame True {
                n114 = invoke class="VI" method="FP.Close"(reference=w300, error in=w301) -> (error out=w302:errorcluster)  [unwired: 1 in, 2 out]
              }
            }
          }
        }
        n115 = call <vilib>:"Add State(s) to Queue__JKI_lib_State_Machine.vi"("State(s) in (\"\")"=w280) -> ("States Out"=w279:string)  [unwired: 14 in]
      }
      frame "---------- Macro ----------" {
        # "Do not put any code in this frame.\n(It is a separator no-op. You can make a copy of this frame to create a new Macro frame)"
        n116 = call <vilib>:"Add State(s) to Queue__JKI_lib_State_Machine.vi"("State(s) in (\"\")"=w306) -> ("States Out"=w305:string)  [unwired: 14 in]
      }
      frame "Macro: Initialize" {
        w307 = "Data: Initialize\nInitialize Core Data\nUI: Initialize\nUI: Front Panel State >> Open"  # Data: Initialize Initialize Core Data UI: Initialize UI: Front Panel State >> Open
        # "Initialization Macro\n(This is called once, when the VI starts)"
        n117 = call <vilib>:"Add State(s) to Queue__JKI_lib_State_Machine.vi"("State(s) in Front (\"\")"=w307, "State(s) in (\"\")"=w311) -> ("States Out"=w310:string)  [unwired: 13 in]
      }
      frame "Macro: Exit" {
        # "Exit Macro\n(This is called once, when the VI exits)"
        n118 = Unbundle By Name(w325) -> ("Core.Close Panel on Exit?"=w324:bool, "Data.Digital Input"=w314:refnum<k21>, "Data.Maintenance"=w317:refnum<k21>, "Data.Digital Output"=w318:refnum<k21>)
        n119 = disable-structure shown="Disabled" {
          disable-tunnel: w318 -> [w338 _]
          disable-tunnel: w317 -> [w334 _]
          disable-tunnel: w316 -> [w331 w341]
          disable-tunnel: [w329 w341] -> w315
          disable-tunnel: w314 -> [w328 _]
          frame Disabled {
            n120 = shared-variable-write(w338, w331, u32[] [0, 0]) -> (w339:refnum<k21>, w336:errorcluster)
            n121 = Close Variable Connection(8:w336, 11:w339) -> (0:w332:errorcluster)
            n122 = shared-variable-write(w334, w332, FALSE) -> (w337:refnum<k21>, w335:errorcluster)
            n123 = Close Variable Connection(8:w335, 11:w337) -> (0:w330:errorcluster)
            n124 = Close Variable Connection(8:w330, 11:w328) -> (0:w329:errorcluster)
          }
          frame Enabled {
          }
        }
        n125 = control-ref of="This VI"() -> (w312:refnum<vi>)
        n126 = invoke class="VI" method="FP.Close"(reference=w312, error in=w315) -> (error out=w313:errorcluster)  [unwired: 1 in, 2 out]
        n127 = Select(t="UI: Front Panel State >> Close", s=w324, f="") -> (s? t:f=w321:string)
        n128 = call <vilib>:"Add State(s) to Queue__JKI_lib_State_Machine.vi"("State(s) in (\"\")"=w321, "State(s) at Back (\"\")"="Data: Cleanup\nExit") -> ("States Out"=w319:string)  [unwired: 13 in]
        n129 = call <vilib>:"Add State(s) to Queue__JKI_lib_State_Machine.vi"("State(s) in Front (\"\")"=w319, "State(s) in (\"\")"=w327) -> ("States Out"=w326:string)  [unwired: 13 in]
      }
      frame "---------- Set -----------" {
      }
      frame "SET DO DATA" {
        n130 = Unbundle By Name(w351) -> ("FPGA VI Reference Out"=w352:refnum<k20>)
        n131 = local read "DO Cluster"() -> (w346:T4)
        n132 = disable-structure shown="Enabled" {
          disable-tunnel: w352 -> [w424 w426]
          disable-tunnel: [w422 w426] -> w349
          disable-tunnel: w348 -> [w421 w425]
          disable-tunnel: [w387 w425] -> w347
          disable-tunnel: w346 -> [w355 _]
          frame Disabled {
            n133 = Unbundle By Name(w355) -> ("0"=w420:bool, "1"=w419:bool, "2"=w418:bool, "3"=w417:bool, "4"=w416:bool, "5"=w415:bool, "6"=w414:bool, "7"=w413:bool, "8"=w412:bool, "9"=w411:bool, "10"=w410:bool, "11"=w409:bool, "12"=w408:bool, "13"=w407:bool, "14"=w406:bool, "15"=w405:bool, "16"=w404:bool, "17"=w403:bool, "18"=w402:bool, "19"=w401:bool, "20"=w400:bool, "21"=w399:bool, "22"=w398:bool, "23"=w397:bool, "24"=w396:bool, "25"=w395:bool, "26"=w394:bool, "27"=w393:bool, "28"=w392:bool, "29"=w391:bool, "30"=w390:bool, "31"=w389:bool)
            n134 = xnode "Read/Write Control"("FPGA VI Reference In"=w424, "error in"=w421, "Mod3/DO0"=w420, "Mod3/DO1"=w419, "Mod3/DO2"=w418, "Mod3/DO3"=w417, "Mod3/DO4"=w416, "Mod3/DO5"=w415, "Mod3/DO6"=w414, "Mod3/DO7"=w413, "Mod3/DO8"=w412, "Mod3/DO9"=w411, "Mod3/DO10"=w410, "Mod3/DO11"=w409, "Mod3/DO12"=w408, "Mod3/DO13"=w407, "Mod3/DO14"=w406, "Mod3/DO15"=w405, "Mod3/DO16"=w404, "Mod3/DO17"=w403, "Mod3/DO18"=w402, "Mod3/DO19"=w401, "Mod3/DO20"=w400, "Mod3/DO21"=w399, "Mod3/DO22"=w398, "Mod3/DO23"=w397, "Mod3/DO24"=w396, "Mod3/DO25"=w395, "Mod3/DO26"=w394, "Mod3/DO27"=w393, "Mod3/DO28"=w392, "Mod3/DO29"=w391, "Mod3/DO30"=w390, "Mod3/DO31"=w389) -> ("FPGA VI Reference Out"=w423:refnum<k20>, "error out"=w388:errorcluster)
            n135 = Unbundle By Name(w355) -> ("32"=w386:bool, "33"=w385:bool, "34"=w384:bool, "35"=w383:bool, "36"=w382:bool, "37"=w381:bool, "38"=w380:bool, "39"=w379:bool, "40"=w378:bool, "41"=w377:bool, "42"=w376:bool, "43"=w375:bool, "44"=w374:bool, "45"=w373:bool, "46"=w372:bool, "47"=w371:bool, "48"=w370:bool, "49"=w369:bool, "50"=w368:bool, "51"=w367:bool, "52"=w366:bool, "53"=w365:bool, "54"=w364:bool, "55"=w363:bool, "56"=w362:bool, "57"=w361:bool, "58"=w360:bool, "59"=w359:bool, "60"=w358:bool, "61"=w357:bool, "62"=w356:bool)
            n136 = xnode "Read/Write Control"("FPGA VI Reference In"=w423, "error in"=w388, "Mod3/DO0"=w386, "Mod3/DO1"=w385, "Mod3/DO2"=w384, "Mod3/DO3"=w383, "Mod3/DO4"=w382, "Mod3/DO5"=w381, "Mod3/DO6"=w380, "Mod3/DO7"=w379, "Mod3/DO8"=w378, "Mod3/DO9"=w377, "Mod3/DO10"=w376, "Mod3/DO11"=w375, "Mod3/DO12"=w374, "Mod3/DO13"=w373, "Mod3/DO14"=w372, "Mod3/DO15"=w371, "Mod3/DO16"=w370, "Mod3/DO17"=w369, "Mod3/DO18"=w368, "Mod3/DO19"=w367, "Mod3/DO20"=w366, "Mod3/DO21"=w365, "Mod3/DO22"=w364, "Mod3/DO23"=w363, "Mod3/DO24"=w362, "Mod3/DO25"=w361, "Mod3/DO26"=w360, "Mod3/DO27"=w359, "Mod3/DO28"=w358, "Mod3/DO29"=w357, "Mod3/DO30"=w356) -> ("FPGA VI Reference Out"=w422:refnum<k20>, "error out"=w387:errorcluster)  [unwired: 1 in]
          }
          frame Enabled {
          }
        }
        n137 = Wait Until Next ms Multiple(millisecond multiple=u32 1) -> ()  [unwired: 1 out]
        n138 = call <vilib>:"Add State(s) to Queue__JKI_lib_State_Machine.vi"("State(s) in (\"\")"=w354) -> ("States Out"=w353:string)  [unwired: 14 in]
        n139 = Bundle By Name(cluster=w351, "FPGA VI Reference Out"=w349) -> (w350:T8)
      }
      frame "SET AO DATA" {
        n140 = Unbundle By Name(w452) -> ("FPGA VI Reference Out"=w451:refnum<k20>)
        n141 = Unbundle By Name("AO Cluster") -> ("AO 1"=w446:dbl, "AO 2"=w445:dbl, "AO 3"=w444:dbl, "AO 4"=w443:dbl, "AO 5"=w442:dbl, "AO 6"=w441:dbl, "AO 7"=w440:dbl, "AO 8"=w439:dbl, "AO 9"=w438:dbl, "AO 10"=w437:dbl, "AO 11"=w436:dbl, "AO 12"=w435:dbl, "AO 13"=w434:dbl, "AO 14"=w433:dbl, "AO 15"=w432:dbl, "AO 16"=w431:dbl, "AO 17"=w430:dbl, "AO 18"=w429:dbl, "AO 19"=w428:dbl, "AO 20"=w427:dbl)
        n142 = disable-structure shown="Disabled" {
          disable-tunnel: w451 -> [w478 w480]
          disable-tunnel: [w477 w480] -> w450
          disable-tunnel: w449 -> [w476 w479]
          disable-tunnel: [w475 w479] -> w448
          disable-tunnel: w446 -> [w474 _]
          disable-tunnel: w445 -> [w473 _]
          disable-tunnel: w444 -> [w472 _]
          disable-tunnel: w443 -> [w471 _]
          disable-tunnel: w442 -> [w470 _]
          disable-tunnel: w441 -> [w469 _]
          disable-tunnel: w440 -> [w468 _]
          disable-tunnel: w439 -> [w467 _]
          disable-tunnel: w438 -> [w466 _]
          disable-tunnel: w437 -> [w465 _]
          disable-tunnel: w436 -> [w464 _]
          disable-tunnel: w435 -> [w463 _]
          disable-tunnel: w434 -> [w462 _]
          disable-tunnel: w433 -> [w461 _]
          disable-tunnel: w432 -> [w460 _]
          disable-tunnel: w431 -> [w459 _]
          disable-tunnel: w430 -> [w458 _]
          disable-tunnel: w429 -> [w457 _]
          disable-tunnel: w428 -> [w456 _]
          disable-tunnel: w427 -> [w455 _]
          frame Disabled {
            n143 = xnode "Read/Write Control"("FPGA VI Reference In"=w478, "error in"=w476, "Mod1/AO0..L"=w474, "Mod1/AO0..R"=w473, "Mod1/AO0..H"=w472, "Mod1/AO0..spare"=w471, "Mod7/Spare1"=w470, "Mod7/Out 1"=w469, "Mod7/Out 2"=w468, "Heater Set point (°C)"=w467, "Cooling  Set point (°C)"=w466, "Mod7/Torque M Set point"=w465, "Mod7/Up M Set point"=w464, "Mod7/Hydraulic pump actuator Soll"=w463, "Mod7/Hydraulic clutch Set point"=w462, "Mod7/Spare2"=w461, "Mod7/Spare 3"=w460, "Mod7/Spare 4"=w459, "Mod7/Spare 5"=w458, "Mod7/Spare 6"=w457, "Mod7/Spare 7"=w456, "Mod7/Spare 8"=w455) -> ("FPGA VI Reference Out"=w477:refnum<k20>, "error out"=w475:errorcluster)
          }
          frame Enabled {
          }
        }
        n144 = Bundle By Name(cluster=w452, "FPGA VI Reference Out"=w450) -> (w453:T8)
      }
      frame "---------- Get ----------" {
      }
      frame "GET DI DATA" {
        n145 = Unbundle By Name(w489) -> ("FPGA VI Reference Out"=w487:refnum<k20>)
        n146 = disable-structure shown="Disabled" {
          disable-tunnel: w487 -> [w560 w561]
          disable-tunnel: w486 -> [w559 w562]
          disable-tunnel: [w558 w562] -> w485
          disable-tunnel: [w557 w561] -> w484
          frame Disabled {
            n147 = xnode "Read/Write Control"("FPGA VI Reference In"=w560, "error in"=w559) -> ("FPGA VI Reference Out"=w557:refnum<k20>, "error out"=w558:errorcluster, "I/O Item"=w556:bool, "I/O Item 2"=w555:bool, "I/O Item 3"=w554:bool, "I/O Item 4"=w553:bool, "I/O Item 5"=w552:bool, "I/O Item 6"=w551:bool, "I/O Item 7"=w550:bool, "I/O Item 8"=w549:bool, "I/O Item 9"=w548:bool, "I/O Item 10"=w547:bool, "I/O Item 11"=w546:bool, "I/O Item 12"=w545:bool, "I/O Item 13"=w544:bool, "I/O Item 14"=w543:bool, "I/O Item 15"=w542:bool, "I/O Item 16"=w541:bool, "I/O Item 17"=w540:bool, "I/O Item 18"=w539:bool, "I/O Item 19"=w538:bool, "I/O Item 20"=w537:bool, "I/O Item 21"=w536:bool, "I/O Item 22"=w535:bool, "I/O Item 23"=w534:bool, "I/O Item 24"=w533:bool, "I/O Item 25"=w532:bool, "I/O Item 26"=w531:bool, "I/O Item 27"=w530:bool, "I/O Item 28"=w529:bool, "I/O Item 29"=w528:bool, "I/O Item 30"=w527:bool, "I/O Item 31"=w526:bool, "I/O Item 32"=w525:bool, "I/O Item 33"=w524:bool, "I/O Item 34"=w523:bool, "I/O Item 35"=w522:bool, "I/O Item 36"=w521:bool, "I/O Item 37"=w520:bool, "I/O Item 38"=w519:bool, "I/O Item 39"=w518:bool, "I/O Item 40"=w517:bool, "I/O Item 41"=w516:bool, "I/O Item 42"=w515:bool, "I/O Item 43"=w514:bool, "I/O Item 44"=w513:bool, "I/O Item 45"=w512:bool, "I/O Item 46"=w511:bool, "I/O Item 47"=w510:bool, "I/O Item 48"=w509:bool, "I/O Item 49"=w508:bool, "I/O Item 50"=w507:bool, "I/O Item 51"=w506:bool, "I/O Item 52"=w505:bool, "I/O Item 53"=w504:bool, "I/O Item 54"=w503:bool, "I/O Item 55"=w502:bool, "I/O Item 56"=w501:bool, "I/O Item 57"=w500:bool, "I/O Item 58"=w499:bool, "I/O Item 59"=w498:bool, "I/O Item 60"=w497:bool, "I/O Item 61"=w496:bool, "I/O Item 62"=w495:bool, "I/O Item 63"=w494:bool, "I/O Item 64"=w493:bool)
            n148 = Bundle(cluster=T5 {"1"=FALSE, "2"=TRUE, "3"=FALSE, "4"=TRUE, "5"=TRUE, "6"=FALSE, "7"=FALSE, "8"=TRUE, "9"=TRUE, "10"=TRUE, "11"=TRUE, "12"=TRUE, "13"=TRUE, "14"=TRUE, "15"=TRUE, "16"=TRUE, "17"=TRUE, "18"=TRUE, "19"=TRUE, "20"=TRUE, "21"=TRUE, "22"=TRUE, "23"=FALSE, "24"=FALSE, "25"=FALSE, "26"=TRUE, "27"=FALSE, "28"=FALSE, "29"=TRUE, "30"=TRUE, "31"=TRUE, "32"=TRUE, "33"=TRUE, "34"=TRUE, "35"=TRUE, "36"=TRUE, "37"=TRUE, "38"=FALSE, "39"=FALSE, "40"=FALSE, "41"=FALSE, "42"=TRUE, "43"=TRUE, "44"=TRUE, "45"=TRUE, "46"=TRUE, "47"=TRUE, "48"=TRUE, "49"=TRUE, "50"=TRUE, "51"=TRUE, "52"=TRUE, "53"=TRUE, "54"=TRUE, "55"=TRUE, "56"=FALSE, "57"=FALSE, "58"=TRUE, "59"=TRUE, "60"=TRUE, "61"=TRUE, "62"=TRUE, "63"=TRUE, "64"=TRUE} ("DI Cluster"), "1"=w556, "2"=w555, "3"=w554, "4"=w553, "5"=w552, "6"=w551, "7"=w550, "8"=w549, "9"=w548, "10"=w547, "11"=w546, "12"=w545, "13"=w544, "14"=w543, "15"=w542, "16"=w541, "17"=w540, "18"=w539, "19"=w538, "20"=w537, "21"=w536, "22"=w535, "23"=w534, "24"=w533, "25"=w532, "26"=w531, "27"=w530, "28"=w529, "29"=w528, "30"=w527, "31"=w526, "32"=w525, "33"=w524, "34"=w523, "35"=w522, "36"=w521, "37"=w520, "38"=w519, "39"=w518, "40"=w517, "41"=w516, "42"=w515, "43"=w514, "44"=w513, "45"=w512, "46"=w511, "47"=w510, "48"=w509, "49"=w508, "50"=w507, "51"=w506, "52"=w505, "53"=w504, "54"=w503, "55"=w502, "56"=w501, "57"=w500, "58"=w499, "59"=w498, "60"=w497, "61"=w496, "62"=w495, "63"=w494, "64"=w493) -> (→"DI Cluster":T5)
          }
          frame Enabled {
          }
        }
        n149 = Bundle By Name(cluster=w489, "FPGA VI Reference Out"=w484) -> (w488:T8)
      }
      frame "GET 9082 AI  DATA" {
        n150 = Unbundle By Name(w569) -> ("FPGA VI Reference Out"=w570:refnum<k20>)
        n151 = disable-structure shown="Enabled" {
          disable-tunnel: w570 -> [w599 w601]
          disable-tunnel: [w598 w601] -> w568
          disable-tunnel: w567 -> [w575 w600]
          disable-tunnel: [w574 w600] -> w566
          disable-tunnel: [w573 _] -> w565
          disable-tunnel: [w572 _] -> w563
          frame Disabled {
            n152 = xnode "9082"("FPGA VI Reference In"=w599, "error in"=w575) -> ("FPGA VI Reference Out"=w598:refnum<k20>, "error out"=w574:errorcluster, "Mod2/Engine Speed Brake L"=w597:fxp<+/-,20,5>, "Mod2/Engine Speed Brake R"=w596:fxp<+/-,20,5>, "Mod2/Engine Speed Brake H"=w595:fxp<+/-,20,5>, "Mod2/Spare"=w594:fxp<+/-,20,5>, "Mod8/Torque Brake L"=w593:fxp<+/-,24,5>, "Mod8/Torque Brake  R"=w592:fxp<+/-,24,5>, "Mod8/Torque Brake H"=w591:fxp<+/-,24,5>, "Mod8/Speed Control"=w590:fxp<+/-,24,5>, "Mod8/spare1"=w589:fxp<+/-,24,5>, "Mod8/Share2"=w588:fxp<+/-,24,5>, "Mod8/Engine Speed Wave Sensor"=w587:fxp<+/-,24,5>, "Mod8/Kal 1 Brake L"=w572:fxp<+/-,24,5>, "Mod8/Kal 2 Brake L"=w586:fxp<+/-,24,5>, "Mod8/Kal 1 Brake R"=w585:fxp<+/-,24,5>, "Mod8/Kal 2 Brake R"=w584:fxp<+/-,24,5>, "Mod8/Kal 1 Brake H"=w583:fxp<+/-,24,5>, "Mod8/Kal 2 Brake H"=w582:fxp<+/-,24,5>, "Mod8/Up M"=w581:fxp<+/-,24,5>, "Mod8/Engine Speed M"=w580:fxp<+/-,24,5>, "Mod8/spare3"=w579:fxp<+/-,24,5>)
            n153 = Build Array(w597, w596, w595, w594, w593, w592, w591, w590, w589, w588, w587, w572, w586, w585, w584, w583, w582, w581, w580, w579) -> (w578:fxp<+/-,24,5>[])
            n154 = Number To Fractional String(number=w578) -> (F-format string=w576:string[])  [unwired: 3 in]
            n155 = Build Array(w576) -> (w577:string[][])
            n156 = Transpose 2D Array(2D array=w577) -> (transposed array=w573:string[][])
          }
          frame Enabled {
          }
        }
        n157 = Absolute Value(x=w563) -> ()  [unwired: 1 out]
        n158 = Bundle By Name(cluster=w569, "FPGA VI Reference Out"=w568, "Analog Data"=w565) -> (w564:T8)
      }
      frame "GET 9148 AI  DATA" {
        n159 = Unbundle By Name(w611) -> ("Analog Data"=w604:string[][], "FPGA VI Reference Out"=w609:refnum<k20>)
        n160 = disable-structure shown="Disabled" {
          disable-tunnel: w609 -> [w628 w754]
          disable-tunnel: w608 -> [w627 w753]
          disable-tunnel: [w626 w754] -> w607
          disable-tunnel: [w625 w753] -> w606
          disable-tunnel: [w623 _] -> w605
          frame Disabled {
            w644 = 24808.0
            n161 = xnode "9148"("FPGA VI Reference In"=w628, "error in"=w627) -> ("FPGA VI Reference Out"=w622:refnum<k20>, "error out"=w621:errorcluster, "Mod7/TC0"=w646:fxp<+/-,24,-2>, "Mod7/TC1"=w651:fxp<+/-,24,-2>, "Mod7/TC2"=w652:fxp<+/-,24,-2>, "Mod7/TC3"=w653:fxp<+/-,24,-2>, "Mod7/TC4"=w658:fxp<+/-,24,-2>, "Mod7/TC5"=w659:fxp<+/-,24,-2>, "Mod7/TC6"=w660:fxp<+/-,24,-2>, "Mod7/TC7"=w661:fxp<+/-,24,-2>, "Mod7/TC8"=w670:fxp<+/-,24,-2>, "Mod7/TC9"=w671:fxp<+/-,24,-2>, "Mod7/TC10"=w672:fxp<+/-,24,-2>, "Mod7/TC11"=w673:fxp<+/-,24,-2>, "Mod7/TC12"=w674:fxp<+/-,24,-2>, "Mod7/TC13"=w675:fxp<+/-,24,-2>, "Mod7/TC14"=w676:fxp<+/-,24,-2>, "Mod7/TC15"=w677:fxp<+/-,24,-2>, "Mod4/AI0"=w619:fxp<+/-,24,-4>, "Mod4/AI1"=w618:fxp<+/-,24,-4>, "Mod4/AI2"=w617:fxp<+/-,24,-4>, "Mod4/AI1"=w616:fxp<+/-,24,-4>, "Mod4/AI0"=w615:fxp<+/-,24,-4>, "Mod7/TC13"=w614:fxp<+/-,24,-2>)
            n162 = Build Array(w614, w614, w614, w614, w614, w614, w614, w614, w614, w614, w614, w614, w614, w614, w614, w614) -> (w620:fxp<+/-,24,-2>[])
            n163 = Build Array(w619, w618, w617, w616, w615, w615, w615, w615, w615, w615, w615, w615, w615, w615, w615, w615) -> (w613:fxp<+/-,24,-4>[])
            n164 = xnode "9148"("FPGA VI Reference In"=w622, "error in"=w621) -> ("FPGA VI Reference Out"=w738:refnum<k20>, "error out"=w739:errorcluster, "Mod1/CH0"=w751:fxp<+/-,32,7>, "Mod1/CH1"=w750:fxp<+/-,32,7>, "Mod1/CH3"=w749:fxp<+/-,32,7>, "Mod1/CH3"=w748:fxp<+/-,32,7>)
            n165 = Multiply(x=w646, y=w644) -> (x*y=w647:dbl)
            n166 = Multiply(x=w651, y=w644) -> (x*y=w648:dbl)
            n167 = Multiply(x=w652, y=w644) -> (x*y=w649:dbl)
            n168 = Multiply(x=w653, y=w644) -> (x*y=w650:dbl)
            n169 = Multiply(x=w658, y=w644) -> (x*y=w657:dbl)
            n170 = Multiply(x=w659, y=w644) -> (x*y=w656:dbl)
            n171 = Multiply(x=w660, y=w644) -> (x*y=w655:dbl)
            n172 = Multiply(x=w661, y=w644) -> (x*y=w654:dbl)
            n173 = Multiply(x=w670, y=w644) -> (x*y=w669:dbl)
            n174 = Multiply(x=w671, y=w644) -> (x*y=w668:dbl)
            n175 = Multiply(x=w672, y=w644) -> (x*y=w667:dbl)
            n176 = Multiply(x=w673, y=w644) -> (x*y=w666:dbl)
            n177 = Multiply(x=w674, y=w644) -> (x*y=w662:dbl)
            n178 = Multiply(x=w675, y=w644) -> (x*y=w663:dbl)
            n179 = Multiply(x=w676, y=w644) -> (x*y=w664:dbl)
            n180 = Multiply(x=w677, y=w644) -> (x*y=w665:dbl)
            n181 = xnode "Read/Write Control"("FPGA VI Reference In"=w738, "error in"=w739) -> ("FPGA VI Reference Out"=w626:refnum<k20>, "error out"=w625:errorcluster, "Mod2/AI0"=w702:fxp<+/-,24,5>, "Mod2/AI1"=w706:fxp<+/-,24,5>, "Mod2/AI2"=w710:fxp<+/-,24,5>, "Mod2/AI3"=w714:fxp<+/-,24,5>, "Mod2/AI4"=w718:fxp<+/-,24,5>, "Mod2/AI5"=w722:fxp<+/-,24,5>, "Mod2/AI6"=w726:fxp<+/-,24,5>, "Mod2/AI7"=w729:fxp<+/-,24,5>, "Mod2/AI8"=w730:fxp<+/-,24,5>, "Mod2/AI9"=w731:fxp<+/-,24,5>, "Mod2/AI10"=w732:fxp<+/-,24,5>, "Mod2/AI11"=w733:fxp<+/-,24,5>, "Mod2/AI12"=w734:fxp<+/-,24,5>, "Mod2/AI13"=w735:fxp<+/-,24,5>, "Mod2/AI14"=w736:fxp<+/-,24,5>, "Mod2/AI15"=w737:fxp<+/-,24,5>)
            n182 = Unbundle By Name("Coolant_In_P 2") -> ("Gain"=w703:fxp<+/-,24,5>, "offset"=w704:fxp<+/-,24,5>)
            n183 = Unbundle By Name("Coolant_Out_P 2") -> ("Gain"=w707:fxp<+/-,24,5>, "offset"=w708:fxp<+/-,24,5>)
            n184 = Unbundle By Name("Exhaust_P 2") -> ("Gain"=w711:fxp<+/-,24,5>, "offset"=w712:fxp<+/-,24,5>)
            n185 = Unbundle By Name("Oil_P 2") -> ("Gain"=w715:fxp<+/-,24,5>, "offset"=w716:fxp<+/-,24,5>)
            n186 = Unbundle By Name("Intercooler_In_P 2") -> ("Gain"=w719:fxp<+/-,24,5>, "offset"=w720:fxp<+/-,24,5>)
            n187 = Unbundle By Name("Intercooler_Out_P 2") -> ("Gain"=w723:fxp<+/-,24,5>, "offset"=w724:fxp<+/-,24,5>)
            n188 = Unbundle By Name("Misc_P 2") -> ("Gain"=w727:fxp<+/-,24,5>, "offset"=w728:fxp<+/-,24,5>)
            n189 = call "Pressure converstion.vi"("Mod2/AI9"=w731, "Mod2/AI8"=w730, "Mod2/AI7"=w729, "Mod2/AI15"=w737, "Mod2/AI10"=w732, "Mod2/AI14"=w736, "Mod2/AI11"=w733, "Mod2/AI12"=w734, "Mod2/AI13"=w735) -> ("P8 toP16"=w740:fxp<+/-,48,10>[])  [unwired: 6 in]
            n190 = Multiply(x=w702, y=w703) -> (x*y=w694:fxp<+/-,48,10>)
            n191 = Multiply(x=w706, y=w707) -> (x*y=w705:fxp<+/-,48,10>)
            n192 = Multiply(x=w710, y=w711) -> (x*y=w709:fxp<+/-,48,10>)
            n193 = Multiply(x=w714, y=w715) -> (x*y=w713:fxp<+/-,48,10>)
            n194 = Multiply(x=w718, y=w719) -> (x*y=w717:fxp<+/-,48,10>)
            n195 = Multiply(x=w722, y=w723) -> (x*y=w721:fxp<+/-,48,10>)
            n196 = Multiply(x=w726, y=w727) -> (x*y=w725:fxp<+/-,48,10>)
            n197 = Add(x=w648, y=23.0) -> (x+y=w679:dbl)
            n198 = Add(x=w656, y=23.0) -> (x+y=w683:dbl)
            n199 = Add(x=w669, y=23.0) -> (x+y=w686:dbl)
            n200 = Add(x=w668, y=23.0) -> (x+y=w687:dbl)
            n201 = Add(x=w666, y=23.0) -> (x+y=w689:dbl)
            n202 = Add(x=w663, y=23.0) -> (x+y=w691:dbl)
            n203 = Add(x=w665, y=23.0) -> (x+y=w693:dbl)
            n204 = Add(x=w694, y=w704) -> (x+y=w747:fxp<+/-,48,10>)
            n205 = Add(x=w705, y=w708) -> (x+y=w746:fxp<+/-,48,10>)
            n206 = Add(x=w709, y=w712) -> (x+y=w745:fxp<+/-,48,10>)
            n207 = Add(x=w713, y=w716) -> (x+y=w744:fxp<+/-,48,10>)
            n208 = Add(x=w717, y=w720) -> (x+y=w743:fxp<+/-,48,10>)
            n209 = Add(x=w721, y=w724) -> (x+y=w742:fxp<+/-,48,10>)
            n210 = Add(x=w725, y=w728) -> (x+y=w741:fxp<+/-,48,10>)
            n211 = Add(x=w647, y=23.0) -> (x+y=w678:dbl)
            n212 = Add(x=w649, y=23.0) -> (x+y=w680:dbl)
            n213 = Add(x=w650, y=23.0) -> (x+y=w681:dbl)
            n214 = Add(x=w657, y=23.0) -> (x+y=w682:dbl)
            n215 = Add(x=w655, y=23.0) -> (x+y=w684:dbl)
            n216 = Add(x=w654, y=23.0) -> (x+y=w685:dbl)
            n217 = Add(x=w667, y=23.0) -> (x+y=w688:dbl)
            n218 = Add(x=w662, y=23.0) -> (x+y=w690:dbl)
            n219 = Add(x=w664, y=23.0) -> (x+y=w692:dbl)
            n220 = Build Array (concatenate)(w751, w750, w749, w748, w747, w746, w745, w744, w743, w742, w741, w740, w613, w613, w678, w679, w680, w681, w682, w683, w684, w685, w686, w687, w688, w689, w690, w691, w692, w693, w620) -> (w624:dbl[])
            n221 = Number To Fractional String(number=w624) -> (F-format string=w752:string[])  [unwired: 3 in]
            n222 = Build Array(w752) -> (w623:string[][])
          }
          frame Enabled {
          }
        }
        n223 = Transpose 2D Array(2D array=w605) -> (transposed array=w603:string[][])
        n224 = Build Array (concatenate)(w604, w603) -> (w602:string[][])
        "ANALOG INPUT" <- w602
        n225 = Bundle By Name(cluster=w611, "FPGA VI Reference Out"=w607, "Analog Data"=w602) -> (w610:T8)
      }
    }
  }
